vi "Main Controller.vi"(8 "Error In":errorcluster) -> (0 "Error Out":errorcluster)   [LabVIEW 2017, in "Main controller.lvlib"]
uses:
  Main controller.lvlib
  CTLs/Params.ctl
  DAQ/Controls/Params.ctl
  DAQ/Controls/DAQ Config.ctl
  DAQ/Controls/DAQ Indicators.ctl
  CTLs/Test Type.ctl
  Shutter Module/Controls/Params.ctl
  Monochromator/Controls/VISA parameters.ctl
  Monochromator/Controls/Params.ctl
  Monochromator/Controls/Type.ctl
  Monochromator/Controls/GratingValues.ctl
  Monochromator/Controls/Grating.ctl
  Monochromator/PTI/Controls/Params.ctl
  Monochromator/Custom Oriel drivers/Controls/Params.ctl
  C:/Project Work/icl-optical-software-rewrite/Optical Software Code Simplified/Modules/Monochromator/Cornerstone.dll
  Monochromator/Cornerstone.dll
  CTLs/Test params.ctl
  CTLs/Test Controls.ctl
  CTLs/Test indicators.ctl
  Scope/Controls/Params.ctl
  Scope/Controls/Models.ctl
  Scope/Controls/TPC.ctl
  Scope/Controls/Channels.ctl
  Trigger/Controls/Params.ctl
  Trigger/Controls/Mode.ctl
  Trigger/Controls/Trigger channels.ctl
  Scope/Controls/Acquisition type.ctl
  Scope/Controls/Record length.ctl
  Scope/Controls/Data.ctl
  Scope/Controls/Channel data.ctl
  Colour Wheel/Controls/Params.ctl
  File IO/Controls/Params.ctl
  CTLs/Commands [enum].ctl
  Events/Controls/Action Refs [enum].ctl
  Shutter Module/Shutter.lvlib
  Monochromator/Monochromator.lvlib
  UI/UI.lvlib
  DAQ/DAQ.lvlib
  Serial comms/Serial comms.lvlib
  Scope/Scope.lvlib
  Trigger/Trigger.lvlib
  File IO/File IO.lvlib
  Colour Wheel/Colour Wheel.lvlib
  Monochromator/Custom Oriel drivers/Oriel (custom drivers).lvlib
  Monochromator/PTI/PTI.lvlib
  Events/Events.lvlib
  Processing/Processing.lvlib
panel:
  out "Current State":T1
  in  "Commands":T1
  out "Standalone":bool
  out "Config out":T2={"DAQ"={"Data"={"Live"={"t0"=timestamp(0 s since 1904-01-01), "dt"=1.0, "Y"=[]}, "Accumulated"={"t0"=timestamp(0 s since 1904-01-01), "dt"=1.0, "Y"=[]}, "Averaged"={"t0"=timestamp(0 s since 1904-01-01), "dt"=1.0, "Y"=[]}, "data array"=[], "live time array"=[], "Live (decimated)"={"t0"=timestamp(0 s since 1904-01-01), "dt"=1.0, "Y"=[]}}, "Config"={"Input Config"=-1, "Card"=enum."USB-6211", "100% Reflectance Standard (V)"=1.0, "Input Channel"="Dev2/ai0", "Average number of points"=10.0, "Trigger Level (V)"=0.3, "Rate (Hz)"=250000, "End Time (s)"=1.0}, "Indicators"={"Final number of points"=0.0, "Number of samples"=0.0, "dt"=0.0, "Shots"=1, "Shot counter"=0, "Test counter"=0, "Background level (V)"=0.0, "DAQ task"="", "timestamp of data"=timestamp(0 s since 1904-01-01), "Test Type"=enum."A-Test"}}, "Shutter"={"Open command string"="", "VISA"={"Timeout (ms)"=0, "Resource Name"="", "Baud Rate"=0, "Data Bits"=0, "Parity"=0, "Stop Bits"=0, "Flow Control"=0}}, "Monochromator"={"Type"=enum."Oriel", "Wavelength (nm)"=0.0, "Grating, gr/mm"=enum."2400", "Grating mode"=enum."Unknown", "Spectrum mode"={"Spectrum mode?"=FALSE, "Start wavelength (nm)"=0.0, "End wavelength (nm)"=0.0, "Wavelength step (nm)"=0.0, "Wavelength array"=[], "array index"=0}, "PTI"={"Delay before read (ms)"=0, "Mono 1"={"Timeout (ms)"=0, "Resource Name"="", "Baud Rate"=0, "Data Bits"=0, "Parity"=0, "Stop Bits"=0, "Flow Control"=0}, "Mono 2"={"Timeout (ms)"=0, "Resource Name"="", "Baud Rate"=0, "Data Bits"=0, "Parity"=0, "Stop Bits"=0, "Flow Control"=0}, "Two PTI Monochromators?"=FALSE}, "Oriel (custom)"={"reference"=refnum}, "Force wavelength confirmation (PTI)?"=FALSE}, "Test"={"Config"={"Amplification Factor"=0.0, "100% Reflectance Standard"=0.0, "Calculation Method"=enum."Reflectance", "Option to discard new data?"=FALSE, "Mode"=enum."Spectrum", "Number of Averages"=0, "B Test?"=FALSE}, "Indicators"={"DAQ Background Level (V)"=0.0, "A-Test Counter"=0, "B-Test Counter"=0, "Type"=enum."A-Test", "Scope Background Level (Amps)"=2.0, "TAS only?"=FALSE}}, "Scope"={"Config"={"VISA Resource"="USB0::0x0699::0x039D::C010764::INSTR", "Model"=enum."DPO 2012B", "Timebase"=0.0004, "Timeout (ms)"=60000, "TAS"={"Vertical Range (V)"=2.0, "Vertical Offset (0.0 divs)"=0.0, "Bandwidth"=0, "Probe Attenuation (10.0)"=1.0, "Vertical Coupling"=1, "Impedance"=0, "Multiplication factor"=1.0, "Channel"=enum."Channel 1"}, "TPC"={"Vertical Range (V)"=2.0, "Vertical Offset (0.0 divs)"=0.0, "Bandwidth"=0, "Probe Attenuation (10.0)"=1.0, "Vertical Coupling"=1, "Impedance"=0, "Multiplication factor"=1.0, "Channel"=enum."None"}, "Trigger"={"Mode"=enum."Laser (TAS)", "Source "=enum."Aux", "PIA"={"Test LEDs"=FALSE, "LED line"="", "LED off (s)"=0.0, "LED on (s)"=0.0}, "Threshold (V)"=0.8}}, "Indicators"={"Setup"={"Final number of points"=0.0, "Pretrigger points"=0.0, "Number of readouts"=0, "Model"={"Acquisition Type"=4, "Record length (points)"=1000, "Averages on scope"=4, "Average number of points"=10.0}}, "Timestamp of Data"=timestamp(0 s since 1904-01-01)}, "Data"={"TPC"={"Live data"={"t0"=timestamp(0 s since 1904-01-01), "dt"=1.0, "Y"=[]}, "Averaged data"={"t0"=timestamp(0 s since 1904-01-01), "dt"=1.0, "Y"=[]}, "Accumulated data"={"t0"=timestamp(0 s since 1904-01-01), "dt"=1.0, "Y"=[]}, "Final data"={"t0"=timestamp(0 s since 1904-01-01), "dt"=1.0, "Y"=[]}}, "TAS"={"Live data"={"t0"=timestamp(0 s since 1904-01-01), "dt"=1.0, "Y"=[]}, "Averaged data"={"t0"=timestamp(0 s since 1904-01-01), "dt"=1.0, "Y"=[]}, "Accumulated data"={"t0"=timestamp(0 s since 1904-01-01), "dt"=1.0, "Y"=[]}, "Final data"={"t0"=timestamp(0 s since 1904-01-01), "dt"=1.0, "Y"=[]}}, "Time arrays"={"Time array (decimated)"=[], "waveform"={"t0"=timestamp(0 s since 1904-01-01), "dt"=1.0, "Y"=[]}}}, "Test"={"Config"={"Amplification Factor"=0.0, "100% Reflectance Standard"=0.0, "Calculation Method"=enum."Reflectance", "Option to discard new data?"=FALSE, "Mode"=enum."Spectrum", "Number of Averages"=100, "B Test?"=FALSE}, "Indicators"={"DAQ Background Level (V)"=2.0, "A-Test Counter"=2, "B-Test Counter"=2, "Type"=enum."A-Test", "Scope Background Level (Amps)"=2.0, "TAS only?"=FALSE}}}, "Colour wheel"={"Reference"=0, "Colour Wheel Wavelengths"=[], "Waveform Index"=0, "COM Port"="", "Enabled?"=FALSE}, "File IO"={"Output Folder"=path "C:/Users/Abigail/Documents/Imperial Optical software/Optical Software Code Simplified/Output", "Error file"=path "C:/Users/Abigail/Documents/Imperial Optical software/Optical Software Code Simplified/Error Log.txt", "Config file"=path "C:/Users/Abigail/Documents/Imperial Optical software/Optical Software Code Simplified/Config.ini", "File prefix"="", "Waveform read"={"t0"=timestamp(0 s since 1904-01-01), "dt"=1.0, "Y"=[]}}} {"Scope"."Test"."Config"."Number of Averages" min=0; "Scope"."Indicators"."Setup"."Model"."Record length (points)" items=["1000"=1, "10,000"=10, "100,000"=100, "1,000,000"=1000, "5,000,000"=5000, "10,000,000"=10000]; "Scope"."Indicators"."Setup"."Model"."Acquisition Type" items=["Sample", "Peak Detect", "Hi Res", "Envelope", "Average"]; "Scope"."Config"."Trigger"."Threshold (V)" format="%#_3f"; "Scope"."Config"."TPC"."Impedance" items=["1M", "75", "50"]; "Scope"."Config"."TPC"."Vertical Coupling" items=["AC", "DC", "Ground"]; "Scope"."Config"."TPC"."Bandwidth" items=["FULL", "250 MHz", "150 MHz", "20 MHz"]; "Scope"."Config"."TAS"."Impedance" items=["1M", "75", "50"]; "Scope"."Config"."TAS"."Vertical Coupling" items=["AC", "DC", "Ground"]; "Scope"."Config"."TAS"."Bandwidth" items=["FULL", "250 MHz", "150 MHz", "20 MHz"]; "Scope"."Config"."Timebase" format="%^#_3e"; "Test"."Config"."Number of Averages" min=0; "Monochromator"."PTI"."Mono 2"."Flow Control" items=["1.0"=10, "1.5"=15, "2.0"=20]; "Monochromator"."PTI"."Mono 2"."Stop Bits" items=["None", "Odd", "Even", "Mark", "Space"]; "Monochromator"."PTI"."Mono 2"."Parity" items=["None", "Odd", "Even", "Mark", "Space"]; "Monochromator"."PTI"."Mono 1"."Flow Control" items=["1.0"=10, "1.5"=15, "2.0"=20]; "Monochromator"."PTI"."Mono 1"."Stop Bits" items=["None", "Odd", "Even", "Mark", "Space"]; "Monochromator"."PTI"."Mono 1"."Parity" items=["None", "Odd", "Even", "Mark", "Space"]; "Shutter"."VISA"."Flow Control" items=["None"=0, "XON/XOFF"=1, "RTS/CTS"=2, "DTR/DSR"=4]; "Shutter"."VISA"."Stop Bits" items=["1.0"=10, "1.5"=15, "2.0"=20]; "Shutter"."VISA"."Parity" items=["None", "Odd", "Even", "Mark", "Space"]; "DAQ"."Config"."Input Config" items=["default"=-1, "RSE"=10083, "NRSE"=10078, "Differential"=10106, "Pseudodifferential"=12529]}
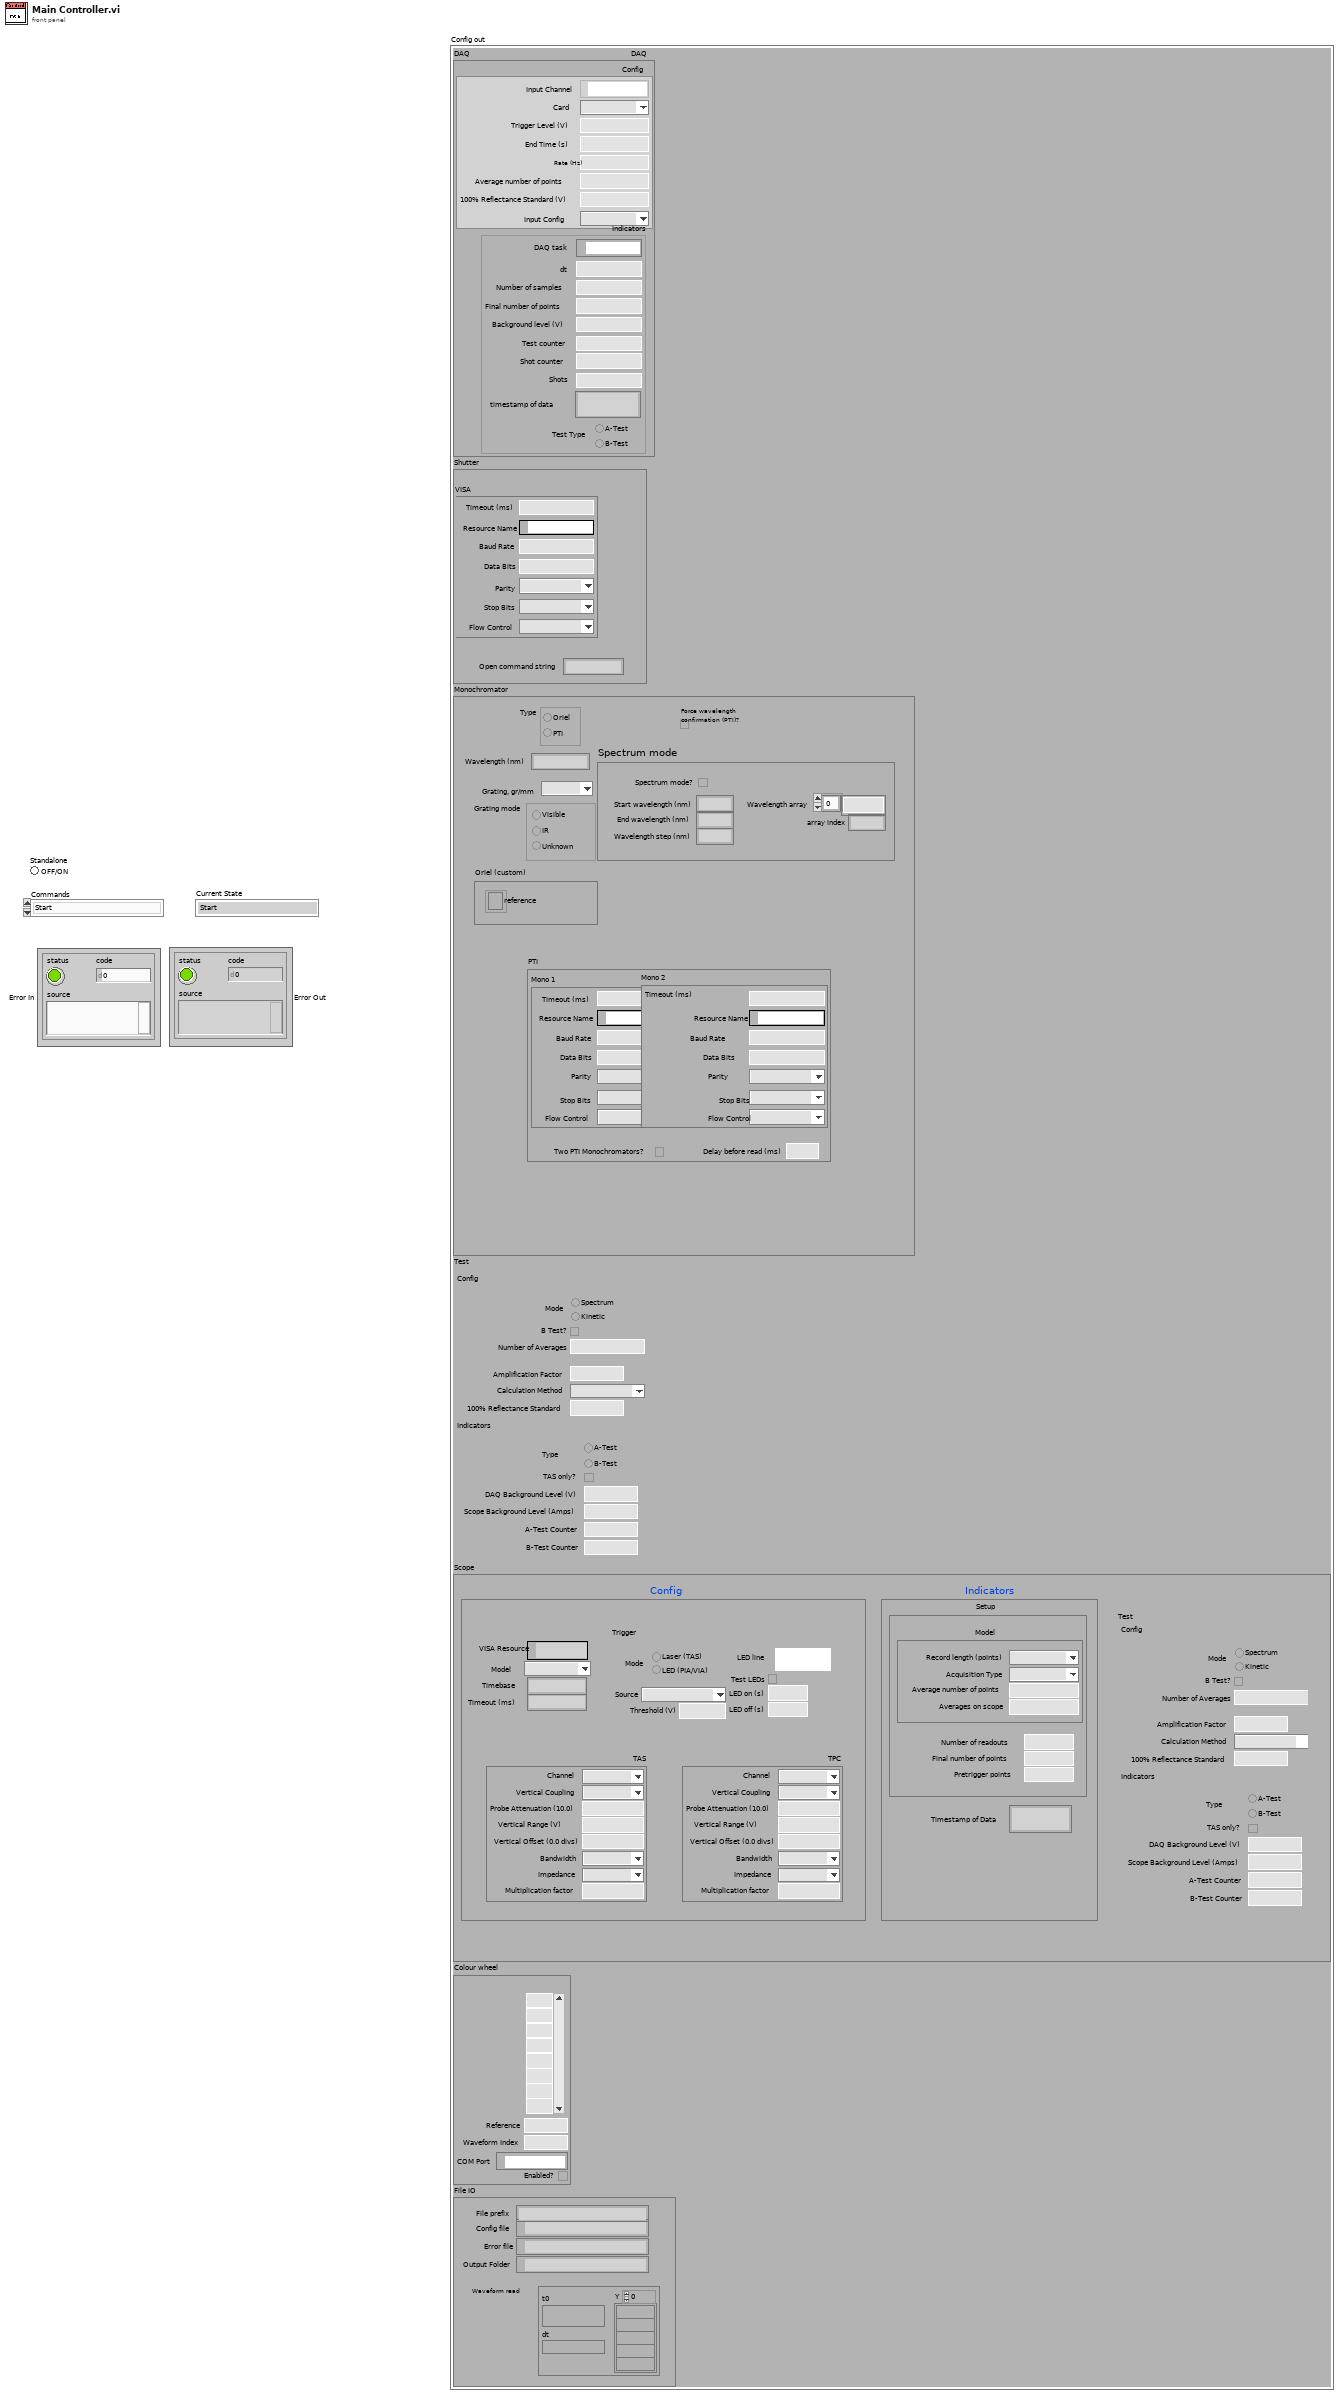
[diagram p1: front panel]
types:
  T1 = typedef "Main controller.lvlib/Commands [enum].ctl" = enum16{"Start", "Initialise Devices", "Stop", "Set DAQ data", "Set Scope data", "Set Spectrum Setup", "Spectrum Setup Complete", "Set Monochromator Setup", "Monochromator Setup Complete", "Set Monochromator data", "Set Colour Wheel Setup", "Colour Wheel Setup Complete", "Move Shutter", "Move Shutter Complete", "Collect Data", "DAQ Acquisition Complete", "Scope Acquisition Complete", "Collect Data Complete", "A-B Processing", "A-B Processing Complete", "DAQ-Scope Stitching", "DAQ-Scope Stitching Complete", "Return Shutter", "Return Shutter Complete", "Set colour wheel data", "Set all config data", "Acquire test data", "Accumulate test data", "Average test data", "All Averaging Complete", "DAQ Averaging Complete", "Scope Averaging Complete", "Finalise test data", "All Finalising Complete", "DAQ Finalising Complete", "Scope Finalising Complete", "Process test data", "End Test"}
  T2 = typedef "Main controller.lvlib/Params.ctl" = cluster{"DAQ":T3, "Shutter":T7, "Monochromator":T9, "Test":T15, "Scope":T18, "Colour wheel":T29, "File IO":T30}
  T3 = typedef "DAQ.lvlib/Params.ctl" = cluster{"Data":cluster{"Live":waveform(dbl), "Accumulated":waveform(dbl), "Averaged":waveform(dbl), "data array":dbl[], "live time array":dbl[], "Live (decimated)":waveform(dbl)}, "Config":T4, "Indicators":T5}
  T4 = typedef "DAQ.lvlib/DAQ Config.ctl" = cluster{"Input Config":i32, "Card":enum16{"USB-6211", "USB-6251", "USB-6361"}, "100% Reflectance Standard (V)":dbl, "Input Channel":tag, "Average number of points":dbl, "Trigger Level (V)":dbl, "Rate (Hz)":i32, "End Time (s)":dbl}
  T5 = typedef "DAQ.lvlib/DAQ Indicators.ctl" = cluster{"Final number of points":dbl, "Number of samples":dbl, "dt":dbl, "Shots":i32, "Shot counter":i32, "Test counter":i32, "Background level (V)":dbl, "DAQ task":refnum<k21>, "timestamp of data":timestamp, "Test Type":T6}
  T6 = typedef "Main controller.lvlib/Test Type.ctl" = enum32{"A-Test", "B-Test"}
  T7 = typedef "Shutter.lvlib/Params.ctl" = cluster{"Open command string":string, "VISA":T8}
  T8 = typedef "Serial comms.lvlib/VISA parameters.ctl" = cluster{"Timeout (ms)":u32, "Resource Name":refnum<visa-resource-name>, "Baud Rate":u32, "Data Bits":u16, "Parity":u16, "Stop Bits":u16, "Flow Control":u16}
  T9 = typedef "Monochromator.lvlib/Params.ctl" = cluster{"Type":T10, "Wavelength (nm)":dbl, "Grating, gr/mm":T11, "Grating mode":T12, "Spectrum mode":cluster{"Spectrum mode?":bool, "Start wavelength (nm)":dbl, "End wavelength (nm)":dbl, "Wavelength step (nm)":dbl, "Wavelength array":dbl[], "array index":u32}, "PTI":T13, "Oriel (custom)":T14, "Force wavelength confirmation (PTI)?":bool}
  T10 = typedef "Monochromator.lvlib/Type.ctl" = enum32{"Oriel", "PTI"}
  T11 = typedef "Monochromator.lvlib/GratingValues.ctl" = enum16{"2400", "1800", "1200", "600", "300", "150"}
  T12 = typedef "Monochromator.lvlib/Grating.ctl" = enum32{"Unknown", "Visible", "IR"}
  T13 = typedef "Monochromator.lvlib/PTI.lvlib/Params.ctl" = cluster{"Delay before read (ms)":u32, "Mono 1":T8, "Mono 2":T8, "Two PTI Monochromators?":bool}
  T14 = typedef "Monochromator.lvlib/Oriel (custom drivers).lvlib/Params.ctl" = cluster{"reference":refnum<k24>}
  T15 = typedef "Main controller.lvlib/Test params.ctl" = cluster{"Config":T16, "Indicators":T17}
  T16 = typedef "Main controller.lvlib/Test Controls.ctl" = cluster{"Amplification Factor":dbl, "100% Reflectance Standard":dbl, "Calculation Method":enum16{"Reflectance", "Transmission", "Kubelka-Munk"}, "Option to discard new data?":bool, "Mode":enum32{"Spectrum", "Kinetic"}, "Number of Averages":i32, "B Test?":bool}
  T17 = typedef "Main controller.lvlib/Test indicators.ctl" = cluster{"DAQ Background Level (V)":dbl, "A-Test Counter":i32, "B-Test Counter":i32, "Type":T6, "Scope Background Level (Amps)":dbl, "TAS only?":bool}
  T18 = typedef "Scope.lvlib/Params.ctl" = cluster{"Config":cluster{"VISA Resource":refnum<visa-resource-name>, "Model":T19, "Timebase":dbl, "Timeout (ms)":u32, "TAS":T20, "TPC":T20, "Trigger":T22}, "Indicators":cluster{"Setup":cluster{"Final number of points":dbl, "Pretrigger points":dbl, "Number of readouts":i32, "Model":cluster{"Acquisition Type":T25, "Record length (points)":T26, "Averages on scope":i32, "Average number of points":dbl}}, "Timestamp of Data":timestamp}, "Data":T27, "Test":T15}
  T19 = typedef "Scope.lvlib/Models.ctl" = enum16{"DPO 3012", "DPO 2012B", "TDS 3012C"}
  T20 = typedef "Scope.lvlib/TPC.ctl" = cluster{"Vertical Range (V)":dbl, "Vertical Offset (0.0 divs)":dbl, "Bandwidth":i32, "Probe Attenuation (10.0)":dbl, "Vertical Coupling":u16, "Impedance":u16, "Multiplication factor":dbl, "Channel":T21}
  T21 = typedef "Scope.lvlib/Channels.ctl" = enum16{"Channel 1", "Channel 2", "Channel 3", "Channel 4", "Math", "Reference A", "Reference B", "Reference C", "Reference D", "B1", "B2", "None"}
  T22 = typedef "Scope.lvlib/Trigger.lvlib/Params.ctl" = cluster{"Mode":T23, "Source ":T24, "PIA":cluster{"Test LEDs":bool, "LED line":tag, "LED off (s)":dbl, "LED on (s)":dbl}, "Threshold (V)":dbl}
  T23 = typedef "Scope.lvlib/Trigger.lvlib/Mode.ctl" = enum32{"Laser (TAS)", "LED (PIA/VIA)"}
  T24 = typedef "Scope.lvlib/Trigger.lvlib/Trigger channels.ctl" = enum16{"Channel 1", "Channel 2", "Channel 3", "Channel 4", "AC Line", "Aux", "Digital Channel 0", "Digital Channel 1", "Digital Channel 2", "Digital Channel 3", "Digital Channel 4", "Digital Channel 5", "Digital Channel 6", "Digital Channel 7", "Digital Channel 8", "Digital Channel 9", "Digital Channel 10", "Digital Channel 11", "Digital Channel 12", "Digital Channel 13", "Digital Channel 14", "Digital Channel 15", "RF"}
  T25 = typedef "Scope.lvlib/Acquisition type.ctl" = u16
  T26 = typedef "Scope.lvlib/Record length.ctl" = u32
  T27 = typedef "Scope.lvlib/Data.ctl" = cluster{"TPC":T28, "TAS":T28, "Time arrays":cluster{"Time array (decimated)":dbl[], "waveform":waveform(dbl)}}
  T28 = typedef "Scope.lvlib/Channel data.ctl" = cluster{"Live data":waveform(dbl), "Averaged data":waveform(dbl), "Accumulated data":waveform(dbl), "Final data":waveform(dbl)}
  T29 = typedef "Colour Wheel.lvlib/Params.ctl" = cluster{"Reference":i32, "Colour Wheel Wavelengths":dbl[], "Waveform Index":i32, "COM Port":refnum<visa-resource-name>, "Enabled?":bool}
  T30 = typedef "File IO.lvlib/Params.ctl" = cluster{"Output Folder":path, "Error file":path, "Config file":path, "File prefix":string, "Waveform read":waveform(dbl)}
  T31 = cluster{"DAQ Acq Complete":bool, "Scope Acq Complete":bool, "DAQ Average Complete":bool, "Scope Average Complete":bool, "DAQ Finalising Complete":bool, "Scope Finalising Complete":bool, "Test Complete":bool}
  T32 = enum32{"Bad", "Idle", "Run top level", "Running"}
  T33 = typedef "Events.lvlib/Action Refs [enum].ctl" = enum16{"Init", "Ref", "Kill"}
  T34 = typedef "Events.lvlib/Refs [cluster].ctl" = cluster{"Exit":refnum<user-event>, "Controller":refnum<user-event>, "System Error":refnum<user-event>, "UI":refnum<user-event>, "Example Module":refnum<user-event>, "Shutter":refnum<user-event>, "Monochromator":refnum<user-event>, "DAQ":refnum<user-event>, "Scope":refnum<user-event>, "Processing":refnum<user-event>, "File IO":refnum<user-event>, "Colour wheel":refnum<user-event>}
  T35 = cluster{"Live":waveform(dbl), "Accumulated":waveform(dbl), "Averaged":waveform(dbl), "data array":dbl[], "live time array":dbl[], "Live (decimated)":waveform(dbl)}
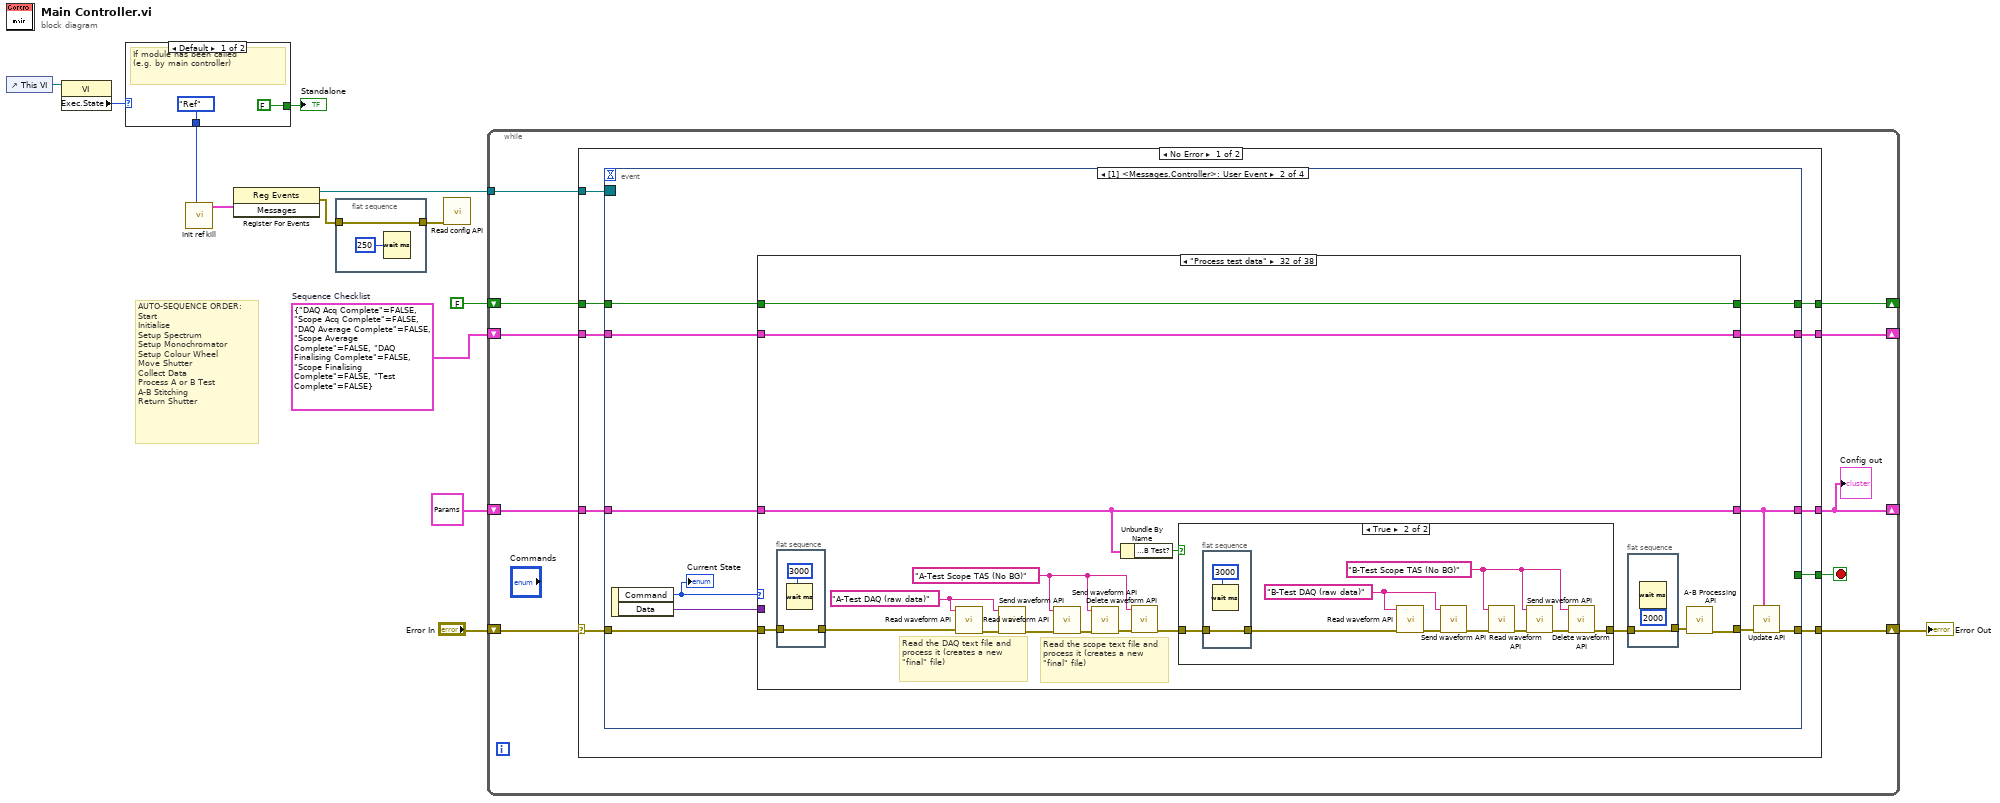
[diagram p0: block diagram]
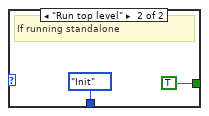
[diagram p2: hidden frame]
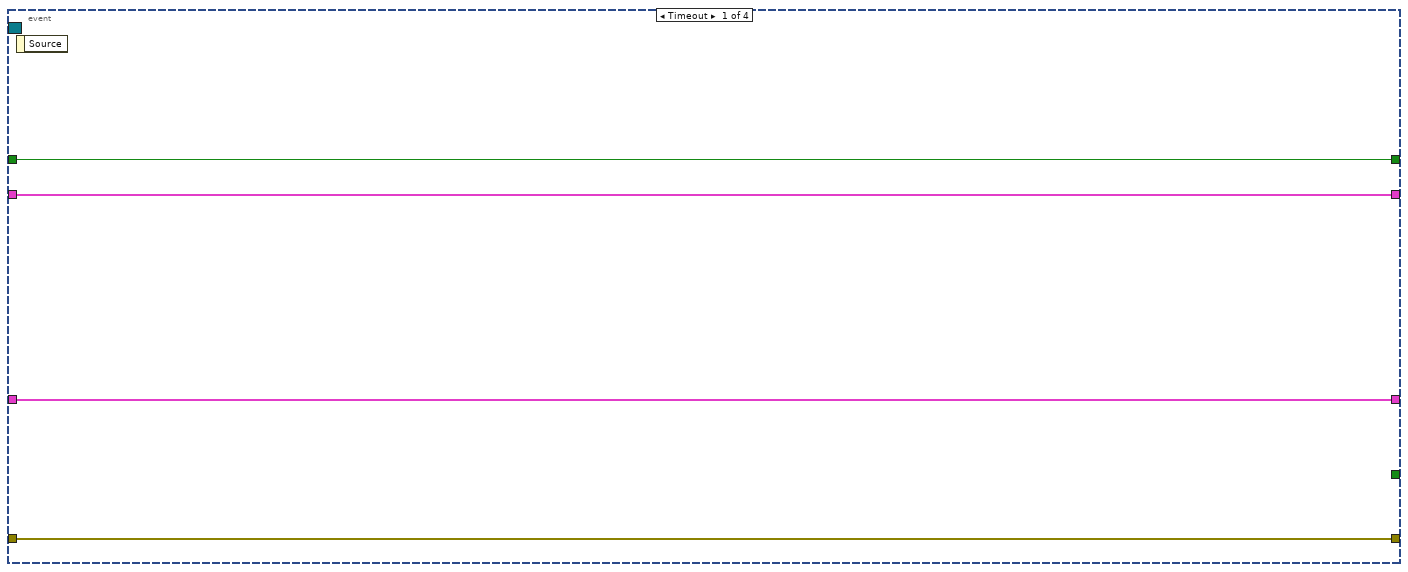
[diagram p3: hidden frame]
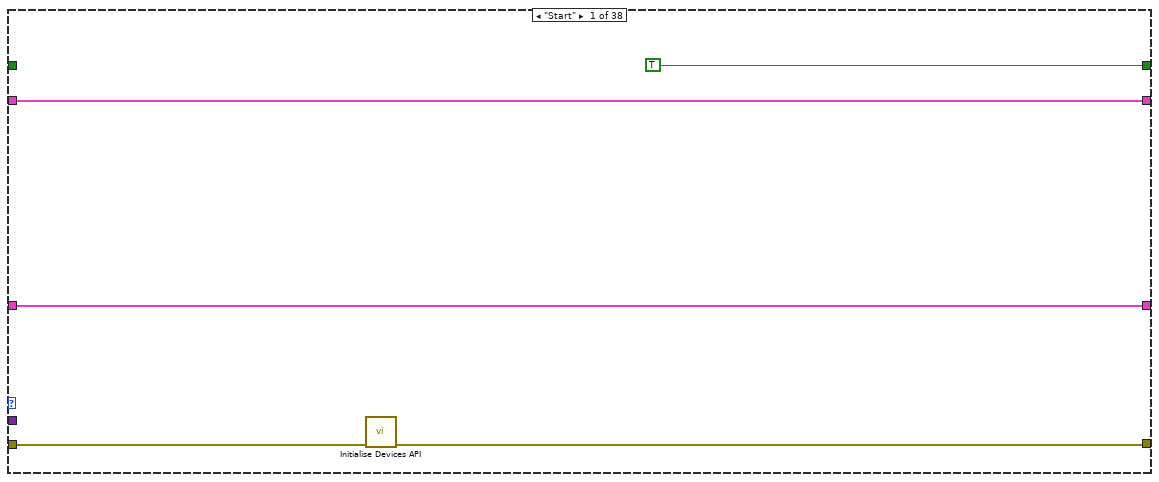
[diagram p4: hidden frame]
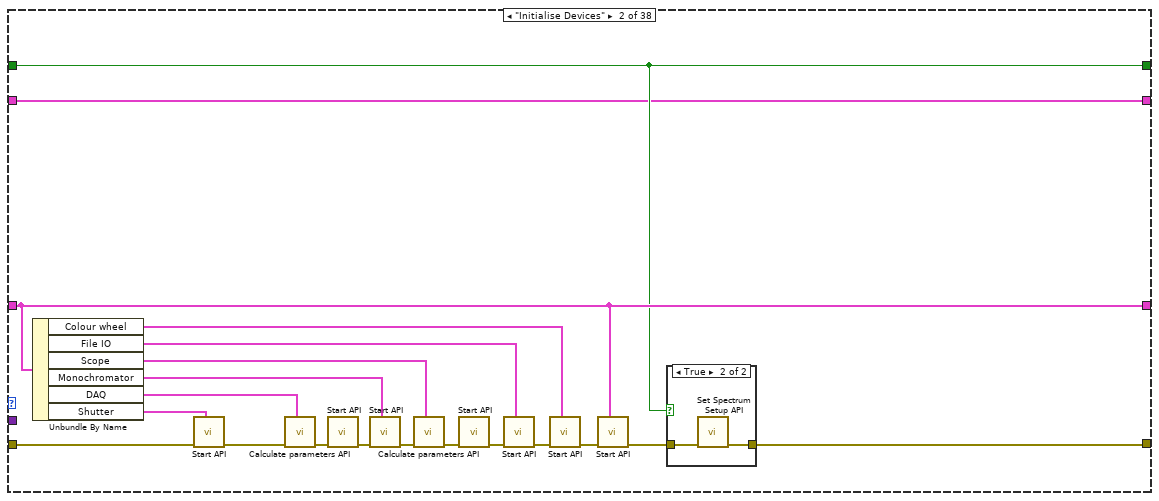
[diagram p5: hidden frame]
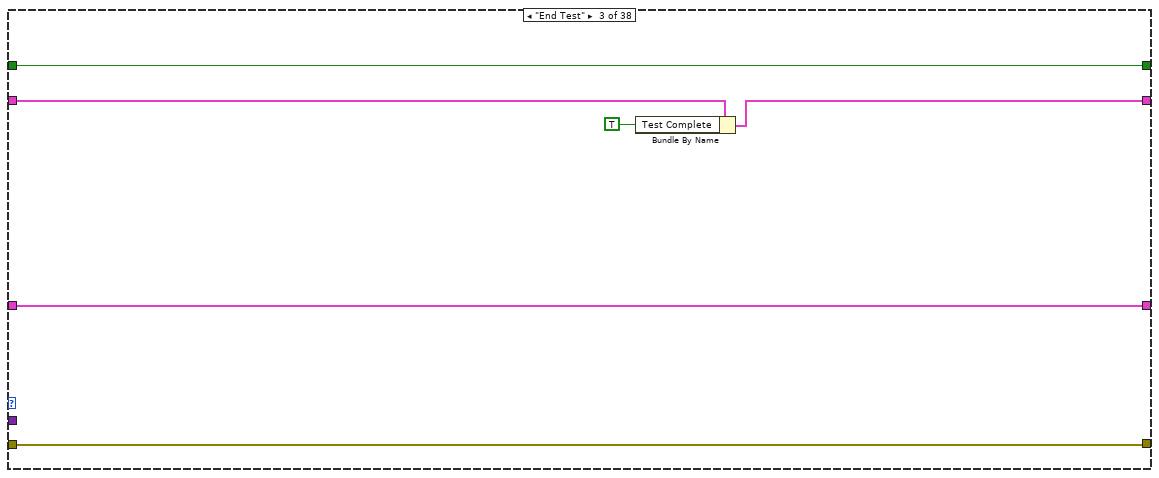
[diagram p7: hidden frame]
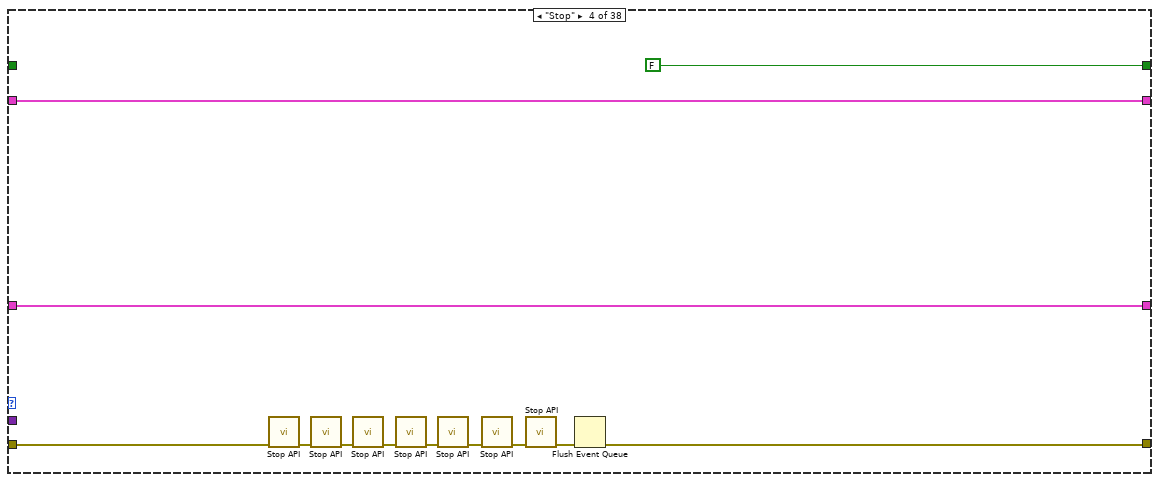
[diagram p8: hidden frame]
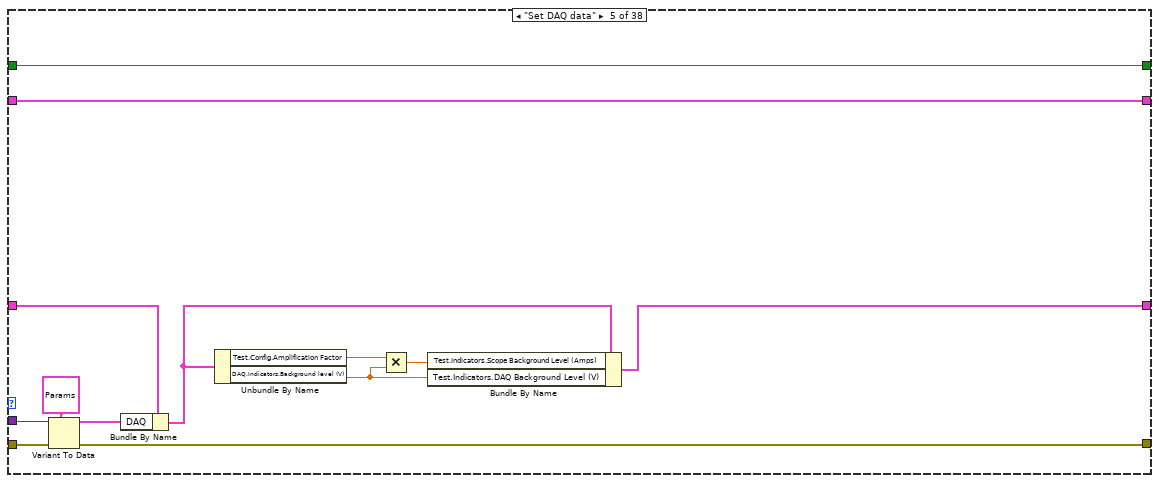
[diagram p9: hidden frame]
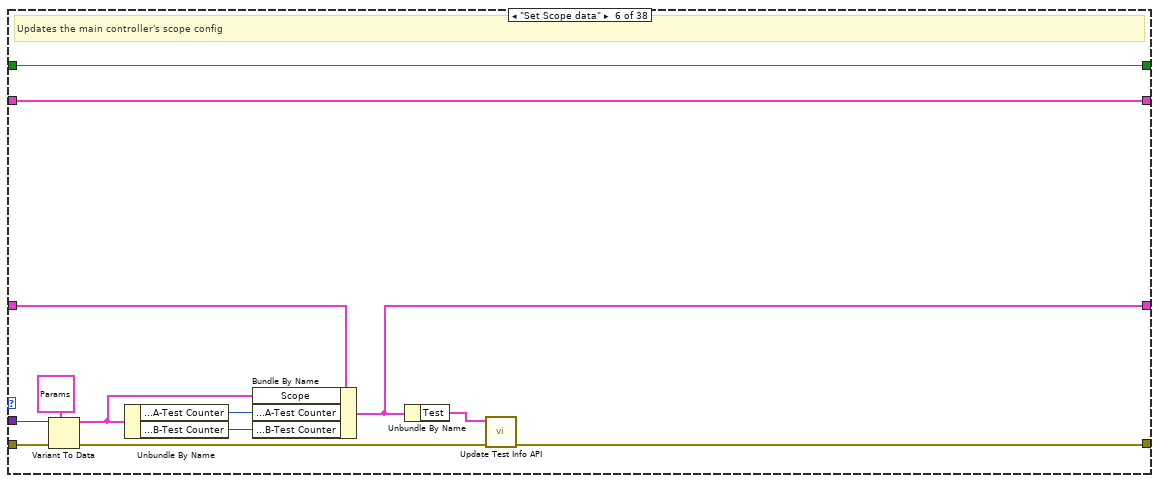
[diagram p10: hidden frame]
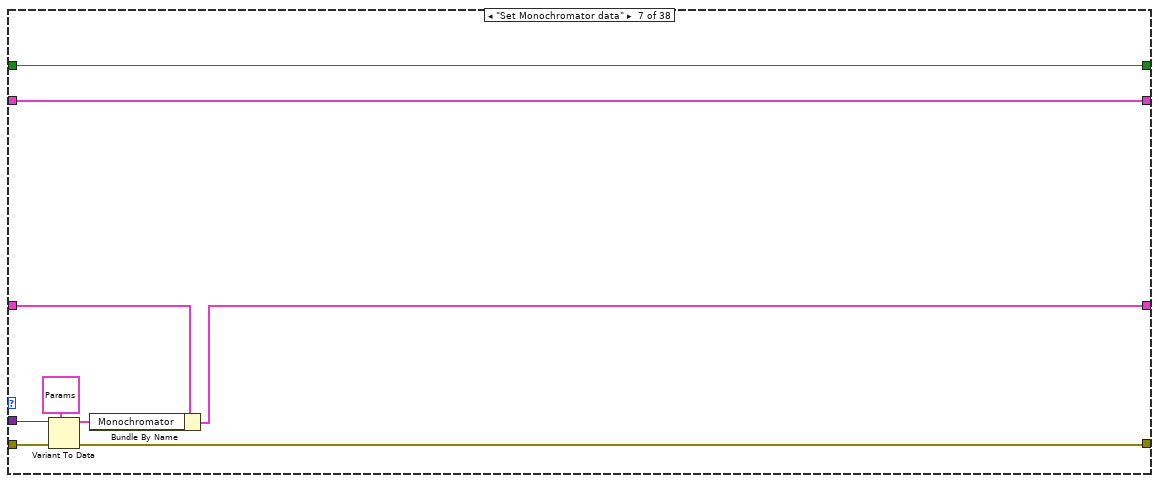
[diagram p11: hidden frame]
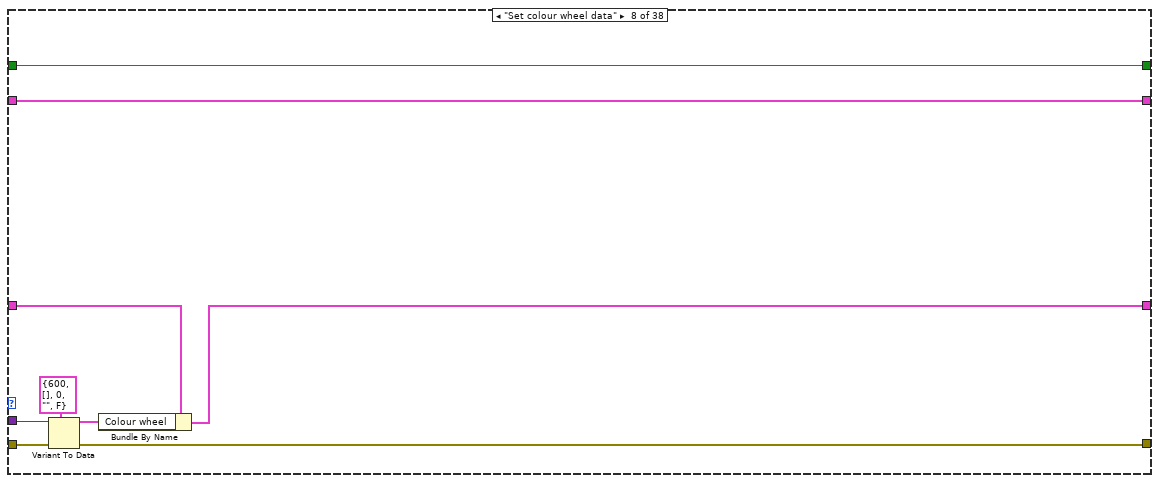
[diagram p12: hidden frame]
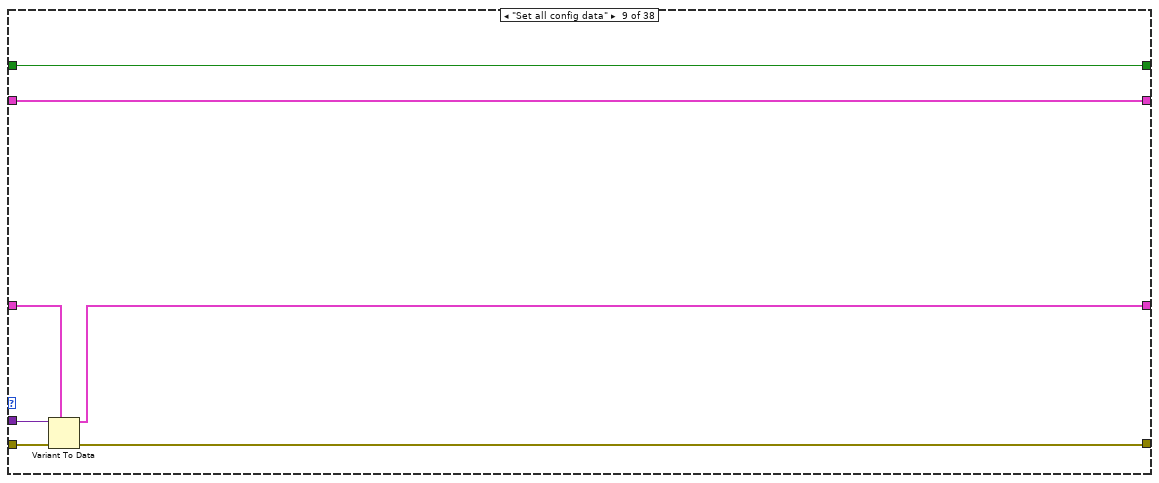
[diagram p13: hidden frame]
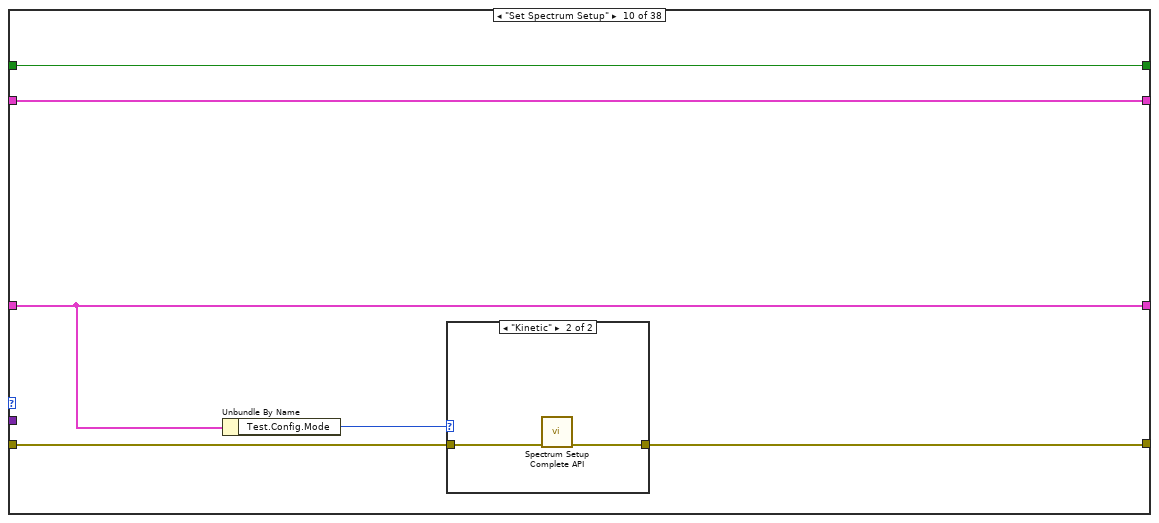
[diagram p14: hidden frame]
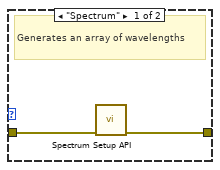
[diagram p15: hidden frame]
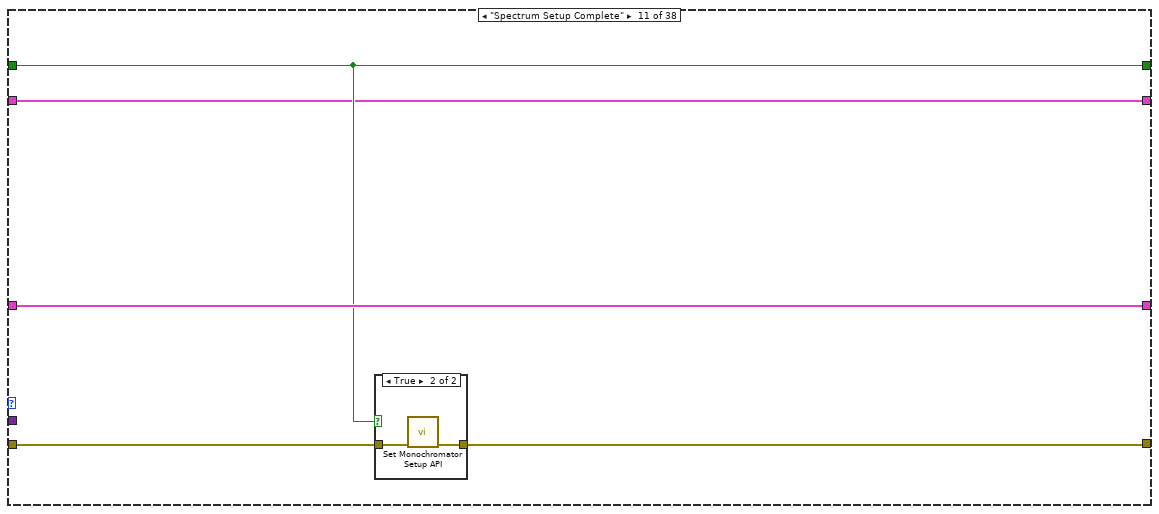
[diagram p16: hidden frame]
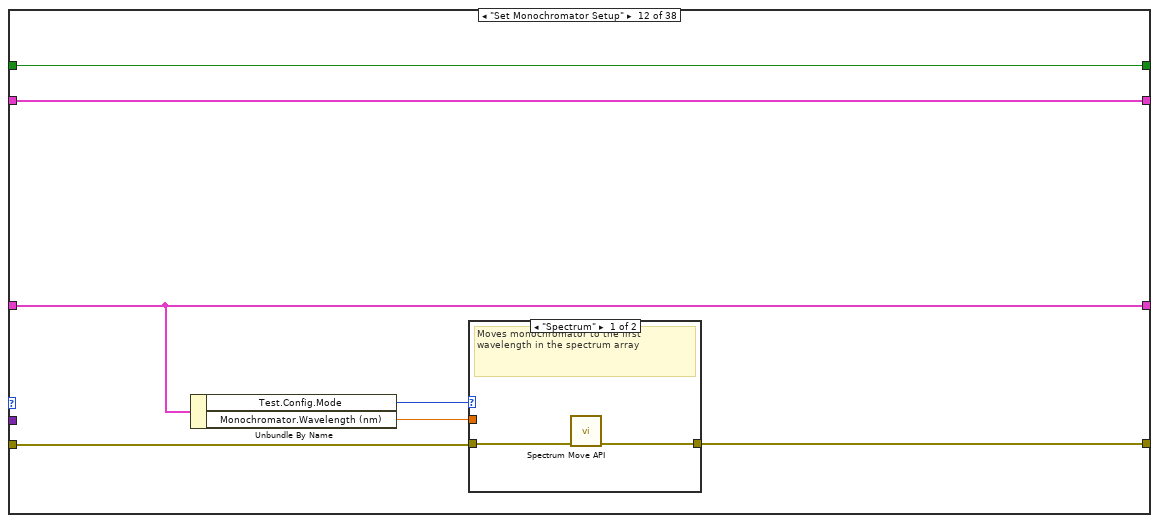
[diagram p18: hidden frame]
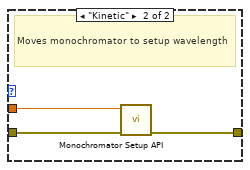
[diagram p19: hidden frame]
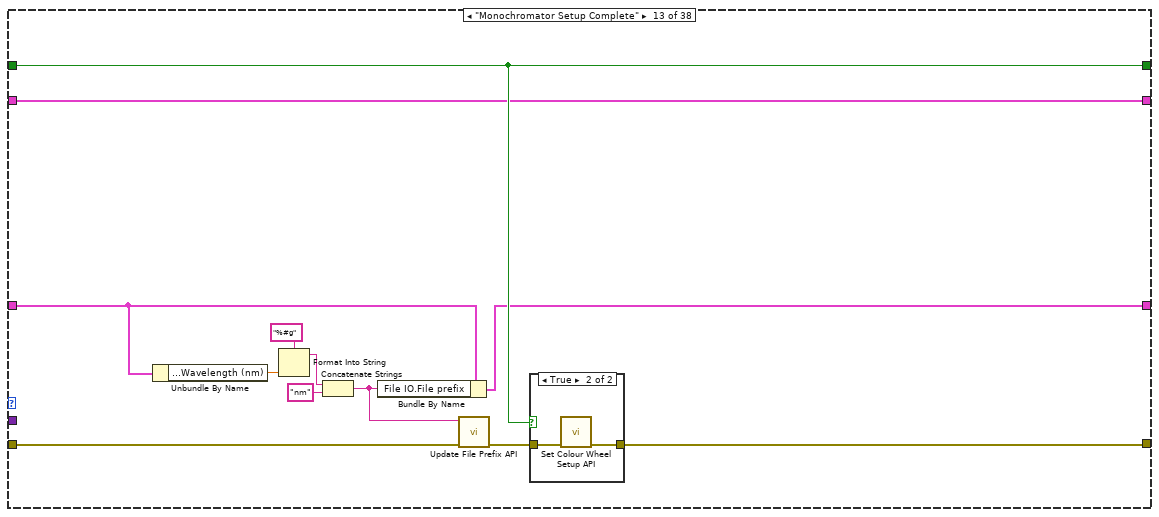
[diagram p20: hidden frame]
diagram:
  w1 = T31 {"DAQ Acq Complete"=FALSE, "Scope Acq Complete"=FALSE, "DAQ Average Complete"=FALSE, "Scope Average Complete"=FALSE, "DAQ Finalising Complete"=FALSE, "Scope Finalising Complete"=FALSE, "Test Complete"=FALSE}  # Sequence Checklist
  # "AUTO-SEQUENCE ORDER:\nStart\nInitialise\nSetup Spectrum\nSetup Monochromator\nSetup Colour Wheel\nMove Shutter\nCollect Data\nProcess A or B Test\nA-B Stitching\nReturn Shutter"
  n1 = control-ref of="This VI"() -> (w11:refnum<vi>)
  n2 = property class="VI"(reference=w11) -> ("Exec.State"=w10:T32)  [unwired: 1 in, 2 out]
  n3 = case shown="Default" w10 {
    tunnel: [Action_Refs_[enum]."Ref" ("Action") Action_Refs_[enum]."Init" ("Action")] -> w9
    tunnel: [FALSE TRUE] -> w8
    frame Default {
      # "If module has been called\n(e.g. by main controller)"
    }
    frame "Run top level" {
      # "If running standalone"
    }
  }
  "Standalone" <- w8
  n4 = call "Init ref kill.vi"("Action"=w9) -> ("Messages"=w5:T34)  [unwired: 9 in, 1 out]
  n5 = register-events(w5) -> (reference out=w4:refnum<event-registration>, error out=w3:errorcluster)  [unwired: 2 in]
  n6 = flat-sequence {
    tunnel: w3 -> [w19]
    tunnel: [w19] -> w2
    frame #0 {
      n7 = Wait (ms)(milliseconds to wait=u32 250) -> ()  [unwired: 1 out]
    }
  }
  n8 = call "Read config API.vi"("Error In"=w2) -> ()  [unwired: 10 in, 1 out]
  n9 = while {
    shift-right: [w29] -> w12
    shift-left: "Error In" -> [w24]
    shift-right: [w26] -> _
    shift-left: T2 {"DAQ"={"Data"={"Live"={"t0"=timestamp(0 s since 1904-01-01), "dt"=1.0, "Y"=[]}, "Accumulated"={"t0"=timestamp(0 s since 1904-01-01), "dt"=1.0, "Y"=[]}, "Averaged"={"t0"=timestamp(0 s since 1904-01-01), "dt"=1.0, "Y"=[]}, "data array"=[], "live time array"=[], "Live (decimated)"={"t0"=timestamp(0 s since 1904-01-01), "dt"=1.0, "Y"=[]}}, "Config"={"Input Config"=10106, "Card"=enum."USB-6211", "100% Reflectance Standard (V)"=1.0, "Input Channel"="Dev1/ai0", "Average number of points"=50.0, "Trigger Level (V)"=0.4, "Rate (Hz)"=250000, "End Time (s)"=1.0}, "Indicators"={"Final number of points"=0.0, "Number of samples"=0.0, "dt"=0.0, "Shots"=1, "Shot counter"=0, "Test counter"=0, "Background level (V)"=0.0, "DAQ task"="", "timestamp of data"=timestamp(0 s since 1904-01-01), "Test Type"=enum."A-Test"}}, "Shutter"={"Open command string"="", "VISA"={"Timeout (ms)"=0, "Resource Name"="", "Baud Rate"=0, "Data Bits"=0, "Parity"=0, "Stop Bits"=0, "Flow Control"=0}}, "Monochromator"={"Type"=enum."Oriel", "Wavelength (nm)"=0.0, "Grating, gr/mm"=enum."2400", "Grating mode"=enum."Unknown", "Spectrum mode"={"Spectrum mode?"=FALSE, "Start wavelength (nm)"=0.0, "End wavelength (nm)"=0.0, "Wavelength step (nm)"=0.0, "Wavelength array"=[], "array index"=0}, "PTI"={"Delay before read (ms)"=0, "Mono 1"={"Timeout (ms)"=0, "Resource Name"="", "Baud Rate"=0, "Data Bits"=0, "Parity"=0, "Stop Bits"=0, "Flow Control"=0}, "Mono 2"={"Timeout (ms)"=0, "Resource Name"="", "Baud Rate"=0, "Data Bits"=0, "Parity"=0, "Stop Bits"=0, "Flow Control"=0}, "Two PTI Monochromators?"=FALSE}, "Oriel (custom)"={"reference"=refnum}, "Force wavelength confirmation (PTI)?"=FALSE}, "Test"={"Config"={"Amplification Factor"=0.0, "100% Reflectance Standard"=0.0, "Calculation Method"=enum."Reflectance", "Option to discard new data?"=FALSE, "Mode"=enum."Spectrum", "Number of Averages"=0, "B Test?"=FALSE}, "Indicators"={"DAQ Background Level (V)"=0.0, "A-Test Counter"=0, "B-Test Counter"=0, "Type"=enum."A-Test", "Scope Background Level (Amps)"=2.0, "TAS only?"=FALSE}}, "Scope"={"Config"={"VISA Resource"="USB0::0x0699::0x039D::C010764::INSTR", "Model"=enum."DPO 2012B", "Timebase"=0.0004, "Timeout (ms)"=60000, "TAS"={"Vertical Range (V)"=2.0, "Vertical Offset (0.0 divs)"=0.0, "Bandwidth"=0, "Probe Attenuation (10.0)"=1.0, "Vertical Coupling"=1, "Impedance"=0, "Multiplication factor"=1.0, "Channel"=enum."Channel 1"}, "TPC"={"Vertical Range (V)"=2.0, "Vertical Offset (0.0 divs)"=0.0, "Bandwidth"=0, "Probe Attenuation (10.0)"=1.0, "Vertical Coupling"=1, "Impedance"=0, "Multiplication factor"=1.0, "Channel"=enum."None"}, "Trigger"={"Mode"=enum."Laser (TAS)", "Source "=enum."Aux", "PIA"={"Test LEDs"=FALSE, "LED line"="", "LED off (s)"=0.0, "LED on (s)"=0.0}, "Threshold (V)"=0.8}}, "Indicators"={"Setup"={"Final number of points"=0.0, "Pretrigger points"=0.0, "Number of readouts"=0, "Model"={"Acquisition Type"=4, "Record length (points)"=1000, "Averages on scope"=4, "Average number of points"=10.0}}, "Timestamp of Data"=timestamp(0 s since 1904-01-01)}, "Data"={"TPC"={"Live data"={"t0"=timestamp(0 s since 1904-01-01), "dt"=1.0, "Y"=[]}, "Averaged data"={"t0"=timestamp(0 s since 1904-01-01), "dt"=1.0, "Y"=[]}, "Accumulated data"={"t0"=timestamp(0 s since 1904-01-01), "dt"=1.0, "Y"=[]}, "Final data"={"t0"=timestamp(0 s since 1904-01-01), "dt"=1.0, "Y"=[]}}, "TAS"={"Live data"={"t0"=timestamp(0 s since 1904-01-01), "dt"=1.0, "Y"=[]}, "Averaged data"={"t0"=timestamp(0 s since 1904-01-01), "dt"=1.0, "Y"=[]}, "Accumulated data"={"t0"=timestamp(0 s since 1904-01-01), "dt"=1.0, "Y"=[]}, "Final data"={"t0"=timestamp(0 s since 1904-01-01), "dt"=1.0, "Y"=[]}}, "Time arrays"={"Time array (decimated)"=[], "waveform"={"t0"=timestamp(0 s since 1904-01-01), "dt"=1.0, "Y"=[]}}}, "Test"={"Config"={"Amplification Factor"=0.0, "100% Reflectance Standard"=0.0, "Calculation Method"=enum."Reflectance", "Option to discard new data?"=FALSE, "Mode"=enum."Spectrum", "Number of Averages"=100, "B Test?"=FALSE}, "Indicators"={"DAQ Background Level (V)"=0.0, "A-Test Counter"=0, "B-Test Counter"=0, "Type"=enum."A-Test", "Scope Background Level (Amps)"=0.0, "TAS only?"=FALSE}}}, "Colour wheel"={"Reference"=0, "Colour Wheel Wavelengths"=[], "Waveform Index"=0, "COM Port"="", "Enabled?"=FALSE}, "File IO"={"Output Folder"=path "C:/Users/Abigail/Documents/Imperial Optical software/Optical Software Code Simplified/Output", "Error file"=path "C:/Users/Abigail/Documents/Imperial Optical software/Optical Software Code Simplified/Error Log.txt", "Config file"=path "C:/Users/Abigail/Documents/Imperial Optical software/Optical Software Code Simplified/Config.ini", "File prefix"="", "Waveform read"={"t0"=timestamp(0 s since 1904-01-01), "dt"=1.0, "Y"=[]}}} ("Config") -> [w27]
    tunnel: w4 -> [w25]
    shift-right: [w22] -> _
    shift-left: FALSE -> [w23]
    shift-right: [w20] -> _
    shift-left: w1 -> [w21]
    stop <- w28 stop-if-true
    n10 = case shown="No Error" w24 {
      selector: w24 -> [w34 w661]
      tunnel: [w39 w660] -> w29
      tunnel: [w38 _] -> w28
      tunnel: w27 -> [w37 w662]
      tunnel: [w36 w662] -> w26
      tunnel: w25 -> [w35 _]
      tunnel: w23 -> [w33 w658]
      tunnel: [w32 w658] -> w22
      tunnel: w21 -> [w31 w657]
      tunnel: [w30 w657] -> w20
      frame No Error {
        n11 = event shown="[1] <Messages.Controller>: User Event" {
          selector: w35 -> [_ _ _ _]
          dyn-events: _ -> [_ _ _ _]
          timeout: _ -> [_ _ _ _]
          tunnel: [w43 w49 w591 w656] -> w39
          tunnel: w34 -> [w43 w54 w590 w656]
          tunnel: [_ _ _ TRUE] -> w38
          tunnel: w37 -> [w42 w51 w588 w654]
          tunnel: [w42 w50 w588 w654] -> w36
          tunnel: w33 -> [w41 w48 w587 w653]
          tunnel: [w41 w47 w587 w653] -> w32
          tunnel: w31 -> [w40 w45 w586 w652]
          tunnel: [w40 w44 w586 w652] -> w30
          event Timeout {
            n12 = event-data() -> ()  [unwired: 1 in, 1 out]
          }
          event User Event {
            n13 = event-data() -> ("Command"=w53:T1, "Data"=w52:variant)  [unwired: 1 in]
            "Current State" <- w53
            n14 = case shown="\"Process test data\"" w53 {
              tunnel: w54 -> [w57 w64 w88 w98 w113 w126 w135 w144 w151 w155 w165 w171 w189 w202 w209 w215 w235 w248 w274 w279 w295 w309 w317 w328 w338 w352 w358 w365 w382 w396 w407 w434 w467 w491 w500 w512 w521 w535]
              tunnel: [w56 w62 w88 w89 w108 w119 w129 w138 w149 w154 w164 w173 w193 w204 w208 w216 w231 w247 w275 w283 w295 w309 w316 w325 w338 w352 w357 w366 w382 w396 w404 w445 w468 w490 w499 w511 w520 w534] -> w46
              tunnel: w52 -> [_ _ _ _ w112 w125 w134 w143 w150 _ _ _ _ _ _ _ _ _ _ _ _ _ _ _ _ _ _ _ _ _ _ _ _ _ _ _ _ _]
              tunnel: w51 -> [w58 w65 w83 w97 w109 w124 w132 w141 w147 w153 w166 w170 w187 w198 w210 w217 w232 w245 w270 w280 w294 w308 w318 w322 w337 w351 w361 w367 w381 w395 w409 w436 w469 w492 w498 w514 w519 w530]
              tunnel: [w58 w65 w83 w97 w103 w117 w131 w140 w148 w153 w166 w170 w186 w198 w210 w217 w232 w246 w270 w280 w294 w308 w318 w322 w337 w351 w361 w367 w381 w395 w408 w436 w469 w492 w498 w514 w519 w529] -> w50
              tunnel: w48 -> [_ w61 w87 _ w107 w122 w128 w137 w146 w157 w163 w176 w192 w205 w207 w220 w234 w250 w272 w282 w293 w307 w315 w324 w336 w350 w360 w370 w380 w394 w411 w444 w471 w489 w502 w510 w523 _]
              tunnel: [TRUE w61 w87 FALSE w107 w122 w128 w137 w146 w157 w163 w176 w192 w205 w207 w220 w234 w250 w272 w282 w293 w307 w315 w324 w336 w350 w360 w370 w380 w394 w411 w444 w471 w489 w502 w510 w523 w531] -> w47
              tunnel: w45 -> [w55 w60 w86 w91 w106 w121 w127 w136 w145 w152 w162 w172 w191 w203 w206 w219 w233 w241 w271 w281 w290 w303 w314 w323 w330 w345 w359 w369 w374 w389 w410 w446 w470 w488 w501 w513 w518 w537]
              tunnel: [w55 w60 w85 w91 w106 w121 w127 w136 w145 w152 w162 w172 w191 w203 w206 w219 w233 w240 w271 w281 w287 w301 w314 w323 w329 w344 w359 w369 w373 w388 w410 w446 w470 w488 w501 w513 w518 w537] -> w44
              frame "Start" {
                n15 = call "Initialise Devices API.vi"("Error In"=w57) -> ("Error Out"=w56:errorcluster)  [unwired: 10 in]
              }
              frame "Initialise Devices" {
                n16 = Unbundle By Name(w65) -> ("Colour wheel"=w73:T29, "File IO"=w70:T30, "Scope"=w77:T18, "Monochromator"=w68:T9, "DAQ"=w76:T3, "Shutter"=w67:T7)
                n17 = call "Start API.vi"("Shutter"=w67, "Error In"=w64) -> ("Error Out"=w74:errorcluster)  [unwired: 9 in]
                n18 = call "Calculate parameters API.vi"("DAQ"=w76, "Error In"=w74) -> ("Error Out"=w75:errorcluster)  [unwired: 9 in]
                n19 = call "Start API.vi"("Error In"=w75) -> ("Error Out"=w66:errorcluster)  [unwired: 10 in]
                n20 = call "Start API.vi"("Monochromator"=w68, "Error In"=w66) -> ("Error Out"=w69:errorcluster)  [unwired: 9 in]
                n21 = call "Calculate parameters API.vi"("Scope"=w77, "Error In"=w69) -> ("Error Out"=w78:errorcluster)  [unwired: 9 in]
                n22 = call "Start API.vi"("Error In"=w78) -> ("Error Out"=w79:errorcluster)  [unwired: 10 in]
                n23 = call "Start API.vi"("File IO parameters"=w70, "Error In"=w79) -> ("Error Out"=w71:errorcluster)  [unwired: 9 in]
                n24 = call "Start API.vi"("Colour wheel"=w73, "Error In"=w71) -> ("Error Out"=w72:errorcluster)  [unwired: 9 in]
                n25 = call "Start API.vi"("Config"=w65, "Error In"=w72) -> ("Error Out"=w63:errorcluster)  [unwired: 9 in]
                n26 = case shown="True" w61 {
                  tunnel: w63 -> [w80 w82]
                  tunnel: [w80 w81] -> w62
                  frame False {
                  }
                  frame True {
                    n27 = call "Set Spectrum Setup API.vi"("Error In"=w82) -> ("Error Out"=w81:errorcluster)  [unwired: 10 in]
                  }
                }
              }
              frame "End Test" {
                n28 = Bundle By Name(cluster=w86, "Test Complete"=TRUE) -> (w85:T31)
              }
              frame "Stop" {
                n29 = call "Stop API.vi"("Error In"=w98) -> ("Error Out"=w100:errorcluster)  [unwired: 10 in]
                n30 = call "Stop API.vi"("Error In"=w100) -> ("Error Out"=w99:errorcluster)  [unwired: 10 in]
                n31 = call "Stop API.vi"("Error In"=w99) -> ("Error Out"=w96:errorcluster)  [unwired: 10 in]
                n32 = call "Stop API.vi"("Error In"=w96) -> ("Error Out"=w95:errorcluster)  [unwired: 10 in]
                n33 = call "Stop API.vi"("Error In"=w95) -> ("Error Out"=w94:errorcluster)  [unwired: 10 in]
                n34 = call "Stop API.vi"("Error In"=w94) -> ("Error Out"=w93:errorcluster)  [unwired: 10 in]
                n35 = call "Stop API.vi"("Error In"=w93) -> ("Error Out"=w90:errorcluster)  [unwired: 10 in]
                n36 = Flush Event Queue(3:w90) -> (11:w89:errorcluster)  [unwired: 5 in, 2 out]
              }
              frame "Set DAQ data" {
                n37 = Variant To Data(error in=w113, type=T3 {"Data"={"Live"={"t0"=timestamp(0 s since 1904-01-01), "dt"=1.0, "Y"=[]}, "Accumulated"={"t0"=timestamp(0 s since 1904-01-01), "dt"=1.0, "Y"=[]}, "Averaged"={"t0"=timestamp(0 s since 1904-01-01), "dt"=1.0, "Y"=[]}, "data array"=[], "live time array"=[], "Live (decimated)"={"t0"=timestamp(0 s since 1904-01-01), "dt"=1.0, "Y"=[]}}, "Config"={"Input Config"=0, "Card"=enum."USB-6211", "100% Reflectance Standard (V)"=0.0, "Input Channel"="Dev1/ai0", "Average number of points"=0.0, "Trigger Level (V)"=0.0, "Rate (Hz)"=0, "End Time (s)"=0.0}, "Indicators"={"Final number of points"=0.0, "Number of samples"=0.0, "dt"=0.0, "Shots"=10, "Shot counter"=10, "Test counter"=10, "Background level (V)"=0.0, "DAQ task"="", "timestamp of data"=timestamp(0 s since 1904-01-01), "Test Type"=enum."A-Test"}} ("DAQ"), Variant=w112) -> (data=w110:T3, error out=w108:errorcluster)
                n38 = Bundle By Name(cluster=w109, "DAQ"=w110) -> (w104:T2)
                n39 = Unbundle By Name(w104) -> ("Test.Config.Amplification Factor"=w105:dbl, "DAQ.Indicators.Background level (V)"=w102:dbl)
                n40 = Multiply(x=w105, y=w102) -> (x*y=w101:dbl)
                n41 = Bundle By Name(cluster=w104, "Test.Indicators.Scope Background Level (Amps)"=w101, "Test.Indicators.DAQ Background Level (V)"=w102) -> (w103:T2)
              }
              frame "Set Scope data" {
                # "Updates the main controller's scope config"
                n42 = Variant To Data(error in=w126, type=T18 {"Config"={"VISA Resource"="COM1", "Model"=enum."DPO 2012B", "Timebase"=0.2, "Timeout (ms)"=0, "TAS"={"Vertical Range (V)"=0.0, "Vertical Offset (0.0 divs)"=0.0, "Bandwidth"=0, "Probe Attenuation (10.0)"=0.0, "Vertical Coupling"=1, "Impedance"=2, "Multiplication factor"=1.0, "Channel"=enum."Channel 1"}, "TPC"={"Vertical Range (V)"=0.2, "Vertical Offset (0.0 divs)"=0.0, "Bandwidth"=0, "Probe Attenuation (10.0)"=0.0, "Vertical Coupling"=1, "Impedance"=1, "Multiplication factor"=2.0, "Channel"=enum."B1"}, "Trigger"={"Mode"=enum."Laser (TAS)", "Source "=enum."Channel 1", "PIA"={"Test LEDs"=FALSE, "LED line"="", "LED off (s)"=0.0, "LED on (s)"=0.0}, "Threshold (V)"=10000.0}}, "Indicators"={"Setup"={"Final number of points"=10000.0, "Pretrigger points"=1000.0, "Number of readouts"=0, "Model"={"Acquisition Type"=2, "Record length (points)"=10, "Averages on scope"=1, "Average number of points"=10000.0}}, "Timestamp of Data"=timestamp(0 s since 1904-01-01)}, "Data"={"TPC"={"Live data"={"t0"=timestamp(0 s since 1904-01-01), "dt"=1.0, "Y"=[]}, "Averaged data"={"t0"=timestamp(0 s since 1904-01-01), "dt"=1.0, "Y"=[]}, "Accumulated data"={"t0"=timestamp(0 s since 1904-01-01), "dt"=1.0, "Y"=[]}, "Final data"={"t0"=timestamp(0 s since 1904-01-01), "dt"=1.0, "Y"=[]}}, "TAS"={"Live data"={"t0"=timestamp(0 s since 1904-01-01), "dt"=1.0, "Y"=[]}, "Averaged data"={"t0"=timestamp(0 s since 1904-01-01), "dt"=1.0, "Y"=[]}, "Accumulated data"={"t0"=timestamp(0 s since 1904-01-01), "dt"=1.0, "Y"=[]}, "Final data"={"t0"=timestamp(0 s since 1904-01-01), "dt"=1.0, "Y"=[]}}, "Time arrays"={"Time array (decimated)"=[], "waveform"={"t0"=timestamp(0 s since 1904-01-01), "dt"=1.0, "Y"=[]}}}, "Test"={"Config"={"Amplification Factor"=2.0, "100% Reflectance Standard"=2.0, "Calculation Method"=enum."Reflectance", "Option to discard new data?"=FALSE, "Mode"=enum."Spectrum", "Number of Averages"=0, "B Test?"=FALSE}, "Indicators"={"DAQ Background Level (V)"=2.0, "A-Test Counter"=2, "B-Test Counter"=2, "Type"=enum."A-Test", "Scope Background Level (Amps)"=2.0, "TAS only?"=FALSE}}} ("Scope"), Variant=w125) -> (data=w118:T18, error out=w120:errorcluster)
                n43 = Unbundle By Name(w118) -> ("Test.Indicators.A-Test Counter"=w115:i32, "Test.Indicators.B-Test Counter"=w114:i32)
                n44 = Bundle By Name(cluster=w124, "Scope"=w118, "Test.Indicators.A-Test Counter"=w115, "Test.Indicators.B-Test Counter"=w114) -> (w117:T2)
                n45 = Unbundle By Name(w117) -> ("Test"=w116:T15)
                n46 = call "Update Test Info API.vi"("Error In"=w120, "Test"=w116) -> ("Error Out"=w119:errorcluster)  [unwired: 9 in]
              }
              frame "Set Monochromator data" {
                n47 = Variant To Data(error in=w135, type=T9 {"Type"=enum."PTI", "Wavelength (nm)"=600.0, "Grating, gr/mm"=enum."1200", "Grating mode"=enum."Unknown", "Spectrum mode"={"Spectrum mode?"=FALSE, "Start wavelength (nm)"=0.0, "End wavelength (nm)"=0.0, "Wavelength step (nm)"=0.0, "Wavelength array"=[], "array index"=0}, "PTI"={"Delay before read (ms)"=50, "Mono 1"={"Timeout (ms)"=1000, "Resource Name"="COM1", "Baud Rate"=9600, "Data Bits"=8, "Parity"=0, "Stop Bits"=10, "Flow Control"=0}, "Mono 2"={"Timeout (ms)"=1000, "Resource Name"="COM1", "Baud Rate"=9600, "Data Bits"=8, "Parity"=0, "Stop Bits"=10, "Flow Control"=0}, "Two PTI Monochromators?"=FALSE}, "Oriel (custom)"={"reference"=refnum}, "Force wavelength confirmation (PTI)?"=FALSE} ("Monochromator"), Variant=w134) -> (data=w133:T9, error out=w129:errorcluster)
                n48 = Bundle By Name(cluster=w132, "Monochromator"=w133) -> (w131:T2)
              }
              frame "Set colour wheel data" {
                n49 = Variant To Data(error in=w144, type=T29 {"Reference"=600, "Colour Wheel Wavelengths"=[], "Waveform Index"=0, "COM Port"="", "Enabled?"=FALSE} ("Colour wheel"), Variant=w143) -> (data=w142:T29, error out=w138:errorcluster)
                n50 = Bundle By Name(cluster=w141, "Colour wheel"=w142) -> (w140:T2)
              }
              frame "Set all config data" {
                n51 = Variant To Data(error in=w151, type=w147, Variant=w150) -> (data=w148:T2, error out=w149:errorcluster)
              }
              frame "Set Spectrum Setup" {
                n52 = Unbundle By Name(w153) -> ("Test.Config.Mode"=w156:enum32{"Spectrum", "Kinetic"})
                n53 = case shown="\"Kinetic\"" w156 {
                  tunnel: [w158 w160] -> w154
                  tunnel: w155 -> [w159 w161]
                  frame "Spectrum" {
                    # "Generates an array of wavelengths"
                    n54 = call "Spectrum Setup API.vi"("Error In"=w159) -> ("Error Out"=w158:errorcluster)  [unwired: 10 in]
                  }
                  frame "Kinetic" {
                    n55 = call "Spectrum Setup Complete API.vi"("Error In"=w161) -> ("Error Out"=w160:errorcluster)  [unwired: 10 in]
                  }
                }
              }
              frame "Spectrum Setup Complete" {
                n56 = case shown="True" w163 {
                  tunnel: w165 -> [w167 w169]
                  tunnel: [w167 w168] -> w164
                  frame False {
                  }
                  frame True {
                    n57 = call "Set Monochromator Setup API.vi"("Error In"=w169) -> ("Error Out"=w168:errorcluster)  [unwired: 10 in]
                  }
                }
              }
              frame "Set Monochromator Setup" {
                n58 = Unbundle By Name(w170) -> ("Test.Config.Mode"=w175:enum32{"Spectrum", "Kinetic"}, "Monochromator.Wavelength (nm)"=w174:dbl)
                n59 = case shown="\"Spectrum\"" w175 {
                  tunnel: [w178 w180] -> w173
                  tunnel: w171 -> [w177 w181]
                  tunnel: w174 -> [_ w179]
                  frame "Spectrum" {
                    # "Moves monochromator to the first wavelength in the spectrum array"
                    n60 = call "Spectrum Move API.vi"("Error In"=w177) -> ("Error Out"=w178:errorcluster)  [unwired: 10 in]
                  }
                  frame "Kinetic" {
                    # "Moves monochromator to setup wavelength"
                    n61 = call "Monochromator Setup API.vi"("Error In"=w181, "wavelength"=w179) -> ("Error Out"=w180:errorcluster)  [unwired: 9 in]
                  }
                }
              }
              frame "Monochromator Setup Complete" {
                n62 = Unbundle By Name(w187) -> ("Monochromator.Wavelength (nm)"=w188:dbl)
                n63 = Format Into String(format string="%#g", w188) -> (resulting string=w183:string)  [unwired: 2 in, 1 out]
                n64 = Concatenate Strings(w183, "nm" ("string")) -> (w182:string)
                n65 = Bundle By Name(cluster=w187, "File IO.File prefix"=w182) -> (w186:T2)
                n66 = call "Update File Prefix API.vi"("Error In"=w189, "File Prefix"=w182) -> ("Error Out"=w190:errorcluster)  [unwired: 9 in]
                n67 = case shown="True" w192 {
                  tunnel: w190 -> [w194 w196]
                  tunnel: [w194 w195] -> w193
                  frame False {
                  }
                  frame True {
                    n68 = call "Set Colour Wheel Setup API.vi"("Error In"=w196) -> ("Error Out"=w195:errorcluster)  [unwired: 10 in]
                  }
                }
              }
              frame "Set Colour Wheel Setup" {
                # "The colour wheel requires the monochromator to spit out its current wavelength before it can move to that wavelength"
                n69 = Unbundle By Name(w198) -> ("Monochromator.Wavelength (nm)"=w200:dbl, "Colour wheel.Colour Wheel Wavelengths"=w197:dbl[])
                n70 = call "Monochromator Wavelength to Colour Wheel Enum.vi"("error in (no error)"=w202, "Possible Wavelengths"=w197, "Wavelength (nm)"=w200) -> ("error out"=w201:errorcluster, "Index"=w199:i32)  [unwired: 7 in]
                n71 = call "Move API.vi"("Error In"=w201, "Index"=w199) -> ("Error Out"=w204:errorcluster)  [unwired: 9 in]
              }
              frame "Colour Wheel Setup Complete" {
                n72 = case shown="True" w207 {
                  tunnel: w209 -> [w211 w213]
                  tunnel: [w211 w212] -> w208
                  frame False {
                  }
                  frame True {
                    n73 = call "Move Shutter API.vi"("Error In"=w213) -> ("Error Out"=w212:errorcluster)  [unwired: 10 in]
                  }
                }
              }
              frame "Move Shutter" {
                n74 = Unbundle By Name(w217) -> ("Test.Config.Mode"=w214:enum32{"Spectrum", "Kinetic"}, "Test.Indicators.Type"=w218:T6)
                n75 = case shown="\"A-Test\"" w218 {
                  tunnel: w215 -> [w224 w230]
                  tunnel: [w221 w229] -> w216
                  tunnel: w214 -> [w223 _]
                  frame "A-Test" {
                    n76 = call "Move Shutter Complete API.vi"("Error In"=w224) -> ("Error Out"=w222:errorcluster)  [unwired: 10 in]
                    n77 = case shown="\"Spectrum\"" w223 {
                      tunnel: w222 -> [w226 w227]
                      tunnel: [w226 w227] -> w221
                      frame "Spectrum" {
                        n78 = Wait (ms)(milliseconds to wait=u32 20000) -> ()  [unwired: 1 out]
                      }
                      frame "Kinetic" {
                      }
                    }
                  }
                  frame "B-Test" {
                    w228 = u32 10000  # Wait (ms)
                    n79 = call "Move API.vi"("Error In"=w230, "Wait (ms)"=w228) -> ("Error Out"=w229:errorcluster)  [unwired: 9 in]
                  }
                }
              }
              frame "Move Shutter Complete" {
                n80 = case shown="True" w234 {
                  tunnel: w235 -> [w236 w238]
                  tunnel: [w236 w237] -> w231
                  frame False {
                  }
                  frame True {
                    n81 = call "Collect Data API.vi"("Error In"=w238) -> ("Error Out"=w237:errorcluster)  [unwired: 10 in]
                  }
                }
              }
              frame "Collect Data" {
                # "#MP Check whether to stop A Test or B Test here"
                # "#MP Check for B-test is now done in \n'All Finalising Complete' case."
                n82 = Unbundle By Name(w245) -> ("Test"=w249:T15, "Test.Indicators.Type"=w239:T6)
                n83 = case shown="\"A-Test\"" w239 {
                  tunnel: w249 -> [w252 w256]
                  tunnel: [w251 w255] -> w244
                  frame "A-Test" {
                    n84 = Unbundle By Name(w252) -> ("Config.Number of Averages"=w253:i32)
                    n85 = call "GetTestCounter.vi"("Test"=w252) -> ("Current test counter"=w254:i32)  [unwired: 10 in]
                    n86 = Greater Or Equal?(x=w254, y=w253) -> (x >= y?=w251:bool)
                  }
                  frame "B-Test" {
                    n87 = call "GetTestCounter.vi"("Test"=w256) -> ("Current test counter"=w258:i32)  [unwired: 10 in]
                    n88 = Unbundle By Name(w256) -> ("Indicators.A-Test Counter"=w257:i32)
                    n89 = Greater Or Equal?(x=w258, y=w257) -> (x >= y?=w255:bool)
                  }
                }
                n90 = Unbundle By Name(w241) -> ("Test Complete"=w242:bool)
                n91 = Or(x=w242, y=w244) -> (x .or. y?=w243:bool)
                n92 = case shown="False" w243 {
                  tunnel: [w260 w267] -> w246
                  tunnel: w245 -> [w260 w267]
                  tunnel: [w261 w268] -> w247
                  tunnel: w248 -> [w262 w269]
                  tunnel: w241 -> [w259 w266]
                  tunnel: [w259 w264] -> w240
                  frame False {
                    # "Continue to get and accumulate data"
                    n93 = call "Acquire DAQ and scope data API.vi"("Error In"=w262) -> ("Error Out"=w263:errorcluster)  [unwired: 10 in]
                    n94 = call "Accumulate test data API.vi"("Error In"=w263) -> ("Error Out"=w261:errorcluster)  [unwired: 10 in]
                  }
                  frame True {
                    # "End of test data acquisition. Time to average, finalise, and process data"
                    n95 = call "Collect Data Complete API.vi"("Error In"=w269) -> ("Error Out"=w268:errorcluster)  [unwired: 10 in]
                    n96 = Bundle By Name(cluster=w266, "Test Complete"=FALSE ("DAQ Acq Complete")) -> (w264:T31)
                  }
                }
              }
              frame "Acquire test data" {
                n97 = Unbundle By Name(w270) -> ("Scope.Indicators.Setup.Model.Averages on scope"=w273:i32)
                n98 = call "Start acquisition API.vi"("Error In"=w274) -> ("Error Out"=w278:errorcluster)  [unwired: 10 in]
                n99 = call "Get test data API.vi"("Error In"=w278) -> ("Error Out"=w277:errorcluster)  [unwired: 10 in]
                n100 = call "Get test data API.vi"("Error In"=w274, "Shots"=w273) -> ("Error Out"=w276:errorcluster)  [unwired: 9 in]
                n101 = Merge Errors(w277, w276) -> (w275:errorcluster)
              }
              frame "Accumulate test data" {
                n102 = call "Accumulate data API.vi"("Error In"=w279) -> ("Error Out"=w284:errorcluster)  [unwired: 10 in]
                n103 = call "Accumulate data API.vi"("Error In"=w279) -> ("Error Out"=w285:errorcluster)  [unwired: 10 in]
                n104 = Merge Errors(w285, w284) -> (w283:errorcluster)
              }
              frame "DAQ Acquisition Complete" {
                n105 = Bundle By Name(cluster=w290, "DAQ Acq Complete"=TRUE) -> (w286:T31)
                n106 = Unbundle By Name(w286) -> ("DAQ Acq Complete"=w291:bool, "Scope Acq Complete"=w288:bool)
                n107 = And(x=w291, y=w288) -> (x .and. y?=w292:bool)
                n108 = case shown="True" w292 {
                  tunnel: [w296 w298] -> w287
                  tunnel: w286 -> [w296 w299]
                  frame False {
                  }
                  frame True {
                    w297 = FALSE ("DAQ Acq Complete")
                    n109 = Bundle By Name(cluster=w299, "DAQ Acq Complete"=w297, "Scope Acq Complete"=w297) -> (w298:T31)
                    n110 = call "Collect Data API.vi"() -> ()  [unwired: 11 in, 1 out]
                  }
                }
              }
              frame "Scope Acquisition Complete" {
                n111 = Bundle By Name(cluster=w303, "Scope Acq Complete"=TRUE ("DAQ Acq Complete")) -> (w302:T31)
                n112 = Unbundle By Name(w302) -> ("DAQ Acq Complete"=w306:bool, "Scope Acq Complete"=w304:bool)
                n113 = And(x=w306, y=w304) -> (x .and. y?=w300:bool)
                n114 = case shown="False" w300 {
                  tunnel: [w310 w312] -> w301
                  tunnel: w302 -> [w310 w313]
                  frame False {
                  }
                  frame True {
                    w311 = FALSE ("Scope Acq Complete")
                    n115 = Bundle By Name(cluster=w313, "DAQ Acq Complete"=w311, "Scope Acq Complete"=w311) -> (w312:T31)
                    n116 = call "Collect Data API.vi"() -> ()  [unwired: 11 in, 1 out]
                  }
                }
              }
              frame "Collect Data Complete" {
                n117 = case shown="True" w315 {
                  tunnel: w317 -> [w319 w321]
                  tunnel: [w319 w320] -> w316
                  frame False {
                  }
                  frame True {
                    n118 = call "Average test data API.vi"("Error In"=w321) -> ("Error Out"=w320:errorcluster)  [unwired: 10 in]
                  }
                }
              }
              frame "Average test data" {
                n119 = call "Average data API.vi"("Error In"=w328) -> ("Error Out"=w326:errorcluster)  [unwired: 10 in]
                n120 = call "Average data API.vi"("Error In"=w328) -> ("Error Out"=w327:errorcluster)  [unwired: 10 in]
                n121 = Merge Errors(w327, w326) -> (w325:errorcluster)
              }
              frame "DAQ Averaging Complete" {
                n122 = Bundle By Name(cluster=w330, "DAQ Average Complete"=TRUE ("DAQ Acq Complete")) -> (w332:T31)
                n123 = Unbundle By Name(w332) -> ("DAQ Average Complete"=w335:bool, "Scope Average Complete"=w333:bool)
                n124 = And(x=w335, y=w333) -> (x .and. y?=w331:bool)
                n125 = case shown="True" w331 {
                  tunnel: [w339 w340] -> w329
                  tunnel: w332 -> [w339 w341]
                  frame False {
                  }
                  frame True {
                    w342 = FALSE ("Scope Average Complete")
                    n126 = Bundle By Name(cluster=w341, "Scope Average Complete"=w342, "DAQ Average Complete"=w342) -> (w340:T31)
                    n127 = call "All Averaging Complete API.vi"() -> ()  [unwired: 11 in, 1 out]
                  }
                }
              }
              frame "Scope Averaging Complete" {
                n128 = Bundle By Name(cluster=w345, "Scope Average Complete"=TRUE ("DAQ Acq Complete")) -> (w346:T31)
                n129 = Unbundle By Name(w346) -> ("DAQ Average Complete"=w349:bool, "Scope Average Complete"=w347:bool)
                n130 = And(x=w349, y=w347) -> (x .and. y?=w343:bool)
                n131 = case shown="False" w343 {
                  tunnel: [w353 w355] -> w344
                  tunnel: w346 -> [w353 w356]
                  frame False {
                  }
                  frame True {
                    w354 = FALSE ("Scope Finalising Complete")
                    n132 = Bundle By Name(cluster=w356, "DAQ Average Complete"=w354, "DAQ Average Complete"=w354) -> (w355:T31)
                    n133 = call "All Averaging Complete API.vi"() -> ()  [unwired: 11 in, 1 out]
                  }
                }
              }
              frame "All Averaging Complete" {
                n134 = call "Finalise test data API.vi"("Error In"=w358) -> ("Error Out"=w357:errorcluster)  [unwired: 10 in]
              }
              frame "Finalise test data" {
                n135 = call "Average Pre Trigger Data API.vi"("Error In"=w365) -> ("Error Out"=w364:errorcluster)  [unwired: 10 in]
                n136 = call "Background voltage API.vi"("Error In"=w364) -> ("Error Out"=w363:errorcluster)  [unwired: 10 in]
                n137 = flat-sequence {
                  tunnel: w363 -> [w371]
                  tunnel: [w371] -> w362
                  frame #0 {
                    n138 = Wait (ms)(milliseconds to wait=u32 200) -> ()  [unwired: 1 out]
                  }
                }
                n139 = call "Add background voltage API.vi"("Error In"=w362) -> ("Error Out"=w368:errorcluster)  [unwired: 10 in]
                n140 = call "Scale TPC API.vi"("Error In"=w368) -> ("Error Out"=w366:errorcluster)  [unwired: 10 in]
              }
              frame "DAQ Finalising Complete" {
                n141 = Bundle By Name(cluster=w374, "DAQ Finalising Complete"=TRUE ("DAQ Acq Complete")) -> (w376:T31)
                n142 = Unbundle By Name(w376) -> ("DAQ Finalising Complete"=w379:bool, "Scope Finalising Complete"=w377:bool)
                n143 = And(x=w379, y=w377) -> (x .and. y?=w375:bool)
                n144 = case shown="False" w375 {
                  tunnel: [w383 w384] -> w373
                  tunnel: w376 -> [w383 w385]
                  frame False {
                  }
                  frame True {
                    w386 = FALSE ("Scope Average Complete")
                    n145 = Bundle By Name(cluster=w385, "DAQ Finalising Complete"=w386, "Scope Finalising Complete"=w386) -> (w384:T31)
                    n146 = call "All Finalise Complete API.vi"() -> ()  [unwired: 11 in, 1 out]
                  }
                }
              }
              frame "Scope Finalising Complete" {
                n147 = Bundle By Name(cluster=w389, "Scope Finalising Complete"=TRUE ("DAQ Acq Complete")) -> (w390:T31)
                n148 = Unbundle By Name(w390) -> ("DAQ Finalising Complete"=w393:bool, "Scope Finalising Complete"=w391:bool)
                n149 = And(x=w393, y=w391) -> (x .and. y?=w387:bool)
                n150 = case shown="True" w387 {
                  tunnel: [w397 w399] -> w388
                  tunnel: w390 -> [w397 w400]
                  frame False {
                  }
                  frame True {
                    w398 = FALSE ("Scope Finalising Complete")
                    n151 = Bundle By Name(cluster=w400, "DAQ Finalising Complete"=w398, "Scope Finalising Complete"=w398) -> (w399:T31)
                    n152 = call "All Finalise Complete API.vi"() -> ()  [unwired: 11 in, 1 out]
                  }
                }
              }
              frame "All Finalising Complete" {
                n153 = Unbundle By Name(w409) -> ("Test.Config.B Test?"=w402:bool, "Test.Indicators.Type"=w405:T6)
                n154 = Equal?(x=w405, y=Test_Type."A-Test" ("Test.Indicators.Type")) -> (x = y?=w403:bool)
                n155 = And(x=w402, y=w403) -> (x .and. y?=w401:bool)
                n156 = case shown="True" w401 {
                  tunnel: w407 -> [w414 w417]
                  tunnel: [w415 w432] -> w404
                  tunnel: w409 -> [w412 w430]
                  tunnel: [w412 w431] -> w408
                  frame False {
                    # "If the current test is B-Test or the user has selected not to run a B test we carry on to the post-processing steps."
                    n157 = call "Save parameters API.vi"("Error In"=w414, "Config"=w412) -> ("Error Out"=w413:errorcluster)  [unwired: 9 in]
                    n158 = call "Process test data API.vi"("Error In"=w413) -> ("Error Out"=w415:errorcluster)  [unwired: 10 in]
                  }
                  frame True {
                    w419 = 0 ("DAQ.Indicators.Shot counter")
                    w425 = Test_Type."B-Test" ("Test.Indicators.Type")
                    # "If the current test is A-Test we want to repeat it but as a B-Test"
                    n159 = Bundle By Name(cluster=w430, "Test.Indicators.Type"=w425, "Scope.Test.Indicators.Type"=w425, "DAQ.Indicators.Test Type"=w425, "DAQ.Indicators.Shot counter"=w419, "DAQ.Indicators.Test counter"=w419, "DAQ.Data"=T35 {"Live"={"t0"=timestamp(0 s since 1904-01-01), "dt"=1.0, "Y"=[]}, "Accumulated"={"t0"=timestamp(0 s since 1904-01-01), "dt"=1.0, "Y"=[]}, "Averaged"={"t0"=timestamp(0 s since 1904-01-01), "dt"=1.0, "Y"=[]}, "data array"=[], "live time array"=[], "Live (decimated)"={"t0"=timestamp(0 s since 1904-01-01), "dt"=1.0, "Y"=[]}} ("Data"), "Scope.Data"=T27 {"TPC"={"Live data"={"t0"=timestamp(0 s since 1904-01-01), "dt"=1.0, "Y"=[]}, "Averaged data"={"t0"=timestamp(0 s since 1904-01-01), "dt"=1.0, "Y"=[]}, "Accumulated data"={"t0"=timestamp(0 s since 1904-01-01), "dt"=1.0, "Y"=[]}, "Final data"={"t0"=timestamp(0 s since 1904-01-01), "dt"=1.0, "Y"=[]}}, "TAS"={"Live data"={"t0"=timestamp(0 s since 1904-01-01), "dt"=1.0, "Y"=[]}, "Averaged data"={"t0"=timestamp(0 s since 1904-01-01), "dt"=1.0, "Y"=[]}, "Accumulated data"={"t0"=timestamp(0 s since 1904-01-01), "dt"=1.0, "Y"=[]}, "Final data"={"t0"=timestamp(0 s since 1904-01-01), "dt"=1.0, "Y"=[]}}, "Time arrays"={"Time array (decimated)"=[], "waveform"={"t0"=timestamp(0 s since 1904-01-01), "dt"=1.0, "Y"=[]}}} ("Data")) -> (w431:T2)
                    n160 = call "Clear Graphs API.vi"("Error In"=w417) -> ("Error Out"=w416:errorcluster)  [unwired: 10 in]
                    n161 = Unbundle By Name(w431) -> ("DAQ"=w420:T3, "Scope"=w427:T18)
                    n162 = call "Stop API.vi"("Error In"=w416) -> ("Error Out"=w429:errorcluster)  [unwired: 10 in]
                    n163 = call "Calculate parameters API.vi"("Scope"=w427, "Error In"=w429) -> ("Error Out"=w428:errorcluster)  [unwired: 9 in]
                    n164 = call "Start API.vi"("Error In"=w428) -> ("Error Out"=w422:errorcluster)  [unwired: 10 in]
                    n165 = call "Stop API.vi"("Error In"=w422) -> ("Error Out"=w423:errorcluster)  [unwired: 10 in]
                    n166 = call "Calculate parameters API.vi"("DAQ"=w420, "Error In"=w423) -> ("Error Out"=w424:errorcluster)  [unwired: 9 in]
                    n167 = call "Start API.vi"("Error In"=w424) -> ("Error Out"=w421:errorcluster)  [unwired: 10 in]
                    n168 = call "Move Shutter API.vi"("Error In"=w421) -> ("Error Out"=w432:errorcluster)  [unwired: 10 in]
                  }
                }
              }
              frame "Process test data" {
                w439 = "A-Test DAQ (raw data)" ("DAQ average file")
                w440 = "A-Test Scope TAS (No BG)" ("DAQ average file")
                # "Read the DAQ text file and process it (creates a new \"final\" file)"
                # "Read the scope text file and process it (creates a new \"final\" file)"
                n169 = flat-sequence {
                  tunnel: w434 -> [w449]
                  tunnel: [w449] -> w433
                  frame #0 {
                    n170 = Wait (ms)(milliseconds to wait=u32 3000) -> ()  [unwired: 1 out]
                  }
                }
                n171 = call "Read waveform API.vi"("Error In"=w433, "Waveform name"=w439) -> ("Error Out"=w443:errorcluster)  [unwired: 9 in]
                n172 = call "Send waveform API.vi"("Error In"=w443, "Waveform name"=w439) -> ("Error Out"=w448:errorcluster)  [unwired: 9 in]
                n173 = call "Read waveform API.vi"("Error In"=w448, "Waveform name"=w440) -> ("Error Out"=w447:errorcluster)  [unwired: 9 in]
                n174 = call "Send waveform API.vi"("Error In"=w447, "Waveform name"=w440) -> ("Error Out"=w442:errorcluster)  [unwired: 9 in]
                n175 = Unbundle By Name(w436) -> ("Test.Config.B Test?"=w435:bool)
                n176 = call "Delete waveform API.vi"("Error In"=w442, "Waveform name"=w440) -> ("Error Out"=w441:errorcluster)  [unwired: 9 in]
                n177 = case shown="True" w435 {
                  tunnel: w441 -> [w451 w453]
                  tunnel: [w451 w457] -> w438
                  frame False {
                  }
                  frame True {
                    w456 = "B-Test DAQ (raw data)" ("DAQ average file")
                    w458 = "B-Test Scope TAS (No BG)" ("DAQ average file")
                    n178 = flat-sequence {
                      tunnel: w453 -> [w461]
                      tunnel: [w461] -> w452
                      frame #0 {
                        n179 = Wait (ms)(milliseconds to wait=u32 3000) -> ()  [unwired: 1 out]
                      }
                    }
                    n180 = call "Read waveform API.vi"("Error In"=w452, "Waveform name"=w456) -> ("Error Out"=w455:errorcluster)  [unwired: 9 in]
                    n181 = call "Send waveform API.vi"("Error In"=w455, "Waveform name"=w456) -> ("Error Out"=w454:errorcluster)  [unwired: 9 in]
                    n182 = call "Read waveform API.vi"("Error In"=w454, "Waveform name"=w458) -> ("Error Out"=w460:errorcluster)  [unwired: 9 in]
                    n183 = call "Send waveform API.vi"("Error In"=w460, "Waveform name"=w458) -> ("Error Out"=w459:errorcluster)  [unwired: 9 in]
                    n184 = call "Delete waveform API.vi"("Error In"=w459, "Waveform name"=w458) -> ("Error Out"=w457:errorcluster)  [unwired: 9 in]
                  }
                }
                n185 = flat-sequence {
                  tunnel: w438 -> [w463]
                  tunnel: [w463] -> w437
                  frame #0 {
                    n186 = Wait (ms)(milliseconds to wait=u32 2000) -> ()  [unwired: 1 out]
                  }
                }
                n187 = call "A-B Processing API.vi"("Error In"=w437) -> ("Error Out"=w445:errorcluster)  [unwired: 10 in]
              }
              frame "A-B Processing" {
                n188 = Unbundle By Name(w469) -> ("File IO"=w465:T30, "Test.Config.B Test?"=w466:bool)
                n189 = case shown="True" w466 {
                  tunnel: [w472 w474] -> w468
                  tunnel: w465 -> [_ w478]
                  tunnel: w467 -> [w473 w481]
                  frame False {
                    n190 = call "A-B Processing Complete API.vi"("Error In"=w473) -> ("Error Out"=w472:errorcluster)  [unwired: 10 in]
                  }
                  frame True {
                    n191 = call "Scope A-B Processing API.vi"("Error In"=w481, "Filename (B)"="B-Test Scope TAS (Pre Trigger Averaged)" ("DAQ average file"), "Filename (A)"="A-Test Scope TAS (Pre Trigger Averaged)" ("DAQ average file"), "File IO"=w478) -> ("Error Out"=w480:errorcluster)  [unwired: 7 in]
                    n192 = flat-sequence {
                      tunnel: w480 -> [w486]
                      tunnel: [w486] -> w479
                      frame #0 {
                        n193 = Wait (ms)(milliseconds to wait=u32 2000) -> ()  [unwired: 1 out]
                      }
                    }
                    n194 = call "DAQ A-B Processing API.vi"("Error In"=w479, "Filename (B)"="B-Test DAQ (raw data)" ("DAQ average file"), "Filename (A)"="A-Test DAQ (raw data)" ("DAQ average file"), "File IO"=w478) -> ("Error Out"=w475:errorcluster)  [unwired: 7 in]
                    n195 = flat-sequence {
                      tunnel: w475 -> [w484]
                      tunnel: [w484] -> w474
                      frame #0 {
                        n196 = Wait (ms)(milliseconds to wait=u32 2000) -> ()  [unwired: 1 out]
                      }
                    }
                  }
                }
              }
              frame "A-B Processing Complete" {
                n197 = case shown="True" w489 {
                  tunnel: w491 -> [w493 w495]
                  tunnel: [w493 w494] -> w490
                  frame False {
                  }
                  frame True {
                    n198 = call "DAQ-Scope Stitching API.vi"("Error In"=w495) -> ("Error Out"=w494:errorcluster)  [unwired: 10 in]
                  }
                }
              }
              frame "DAQ-Scope Stitching" {
                n199 = Unbundle By Name(w498) -> ("Test.Config.B Test?"=w496:bool, "File IO"=w497:T30)
                n200 = case shown="True" w496 {
                  tunnel: w500 -> [w504 w509]
                  tunnel: [w503 w508] -> w499
                  tunnel: w497 -> [_ w507]
                  frame False {
                    n201 = call "DAQ-Scope Stitching Complete API.vi"("Error In"=w504) -> ("Error Out"=w503:errorcluster)  [unwired: 10 in]
                  }
                  frame True {
                    n202 = call "DAQ-Scope Stitching API.vi"("Error In"=w509, "Scope Filename"="Scope TAS (final A-B)" ("Filename (A)"), "DAQ Filename"="A-Test DAQ (final)" ("Filename (A)"), "File IO"=w507) -> ("Error Out"=w508:errorcluster)  [unwired: 7 in]
                  }
                }
              }
              frame "DAQ-Scope Stitching Complete" {
                n203 = case shown="True" w510 {
                  tunnel: w512 -> [w515 w517]
                  tunnel: [w515 w516] -> w511
                  frame False {
                  }
                  frame True {
                    n204 = call "Return Shutter API.vi"("Error In"=w517) -> ("Error Out"=w516:errorcluster)  [unwired: 10 in]
                  }
                }
              }
              frame "Return Shutter" {
                n205 = Unbundle By Name(w519) -> ("Test.Indicators.Type"=w522:T6)
                n206 = case shown="\"B-Test\"" w522 {
                  tunnel: w521 -> [w525 w528]
                  tunnel: [w524 w527] -> w520
                  frame "A-Test" {
                    n207 = call "Return Shutter Complete API.vi"("Error In"=w525) -> ("Error Out"=w524:errorcluster)  [unwired: 10 in]
                  }
                  frame "B-Test" {
                    n208 = call "Return API.vi"("Error In"=w528, "Wait (ms)"=u32 10000) -> ("Error Out"=w527:errorcluster)  [unwired: 9 in]
                  }
                }
              }
              frame "Return Shutter Complete" {
                # "Keeps a track of wavelengths left to move to so we know \nwhen the Spectrum sequence is complete and we can STOP."
                n209 = Unbundle By Name(w530) -> ("Monochromator.Spectrum mode.array index"=w532:u32, "Monochromator.Spectrum mode.Wavelength array"=w533:dbl[], "Test.Config.Mode"=w536:enum32{"Spectrum", "Kinetic"})
                n210 = case shown="\"Spectrum\"" w536 {
                  tunnel: w535 -> [w546 w580]
                  tunnel: [w545 w582] -> w534
                  tunnel: w533 -> [w544 _]
                  tunnel: w532 -> [w543 _]
                  tunnel: [w540 FALSE] -> w531
                  tunnel: w530 -> [w539 w578]
                  tunnel: [w538 w577] -> w529
                  frame "Spectrum" {
                    n211 = Array Size(array=w544) -> (size(s)=w542:i32)
                    n212 = Greater Or Equal?(x=w543, y=w542) -> (x >= y?=w541:bool)
                    n213 = case shown="True" w541 {
                      tunnel: w546 -> [w552 w569]
                      tunnel: [w565 w572] -> w545
                      tunnel: [TRUE FALSE] -> w540
                      tunnel: w539 -> [w554 w570]
                      tunnel: [w553 w570] -> w538
                      frame False {
                        w550 = T17 {"DAQ Background Level (V)"=0.0, "A-Test Counter"=0, "B-Test Counter"=0, "Type"=enum."A-Test", "Scope Background Level (Amps)"=0.0, "TAS only?"=FALSE} ("Test.Indicators")
                        n214 = Bundle By Name(cluster=w554, "Scope.Test.Indicators"=w550, "Test.Indicators"=w550, "DAQ.Indicators.Test Type"=Test_Type."A-Test", "DAQ.Data"=T35 {"Live"={"t0"=timestamp(0 s since 1904-01-01), "dt"=1.0, "Y"=[]}, "Accumulated"={"t0"=timestamp(0 s since 1904-01-01), "dt"=1.0, "Y"=[]}, "Averaged"={"t0"=timestamp(0 s since 1904-01-01), "dt"=1.0, "Y"=[]}, "data array"=[], "live time array"=[], "Live (decimated)"={"t0"=timestamp(0 s since 1904-01-01), "dt"=1.0, "Y"=[]}} ("Data"), "Scope.Data"=T27 {"TPC"={"Live data"={"t0"=timestamp(0 s since 1904-01-01), "dt"=1.0, "Y"=[]}, "Averaged data"={"t0"=timestamp(0 s since 1904-01-01), "dt"=1.0, "Y"=[]}, "Accumulated data"={"t0"=timestamp(0 s since 1904-01-01), "dt"=1.0, "Y"=[]}, "Final data"={"t0"=timestamp(0 s since 1904-01-01), "dt"=1.0, "Y"=[]}}, "TAS"={"Live data"={"t0"=timestamp(0 s since 1904-01-01), "dt"=1.0, "Y"=[]}, "Averaged data"={"t0"=timestamp(0 s since 1904-01-01), "dt"=1.0, "Y"=[]}, "Accumulated data"={"t0"=timestamp(0 s since 1904-01-01), "dt"=1.0, "Y"=[]}, "Final data"={"t0"=timestamp(0 s since 1904-01-01), "dt"=1.0, "Y"=[]}}, "Time arrays"={"Time array (decimated)"=[], "waveform"={"t0"=timestamp(0 s since 1904-01-01), "dt"=1.0, "Y"=[]}}} ("Data")) -> (w553:T2)
                        n215 = call "Clear Graphs API.vi"("Error In"=w552) -> ("Error Out"=w551:errorcluster)  [unwired: 10 in]
                        n216 = Unbundle By Name(w553) -> ("DAQ"=w557:T3, "Scope"=w563:T18)
                        n217 = call "Stop API.vi"("Error In"=w551) -> ("Error Out"=w561:errorcluster)  [unwired: 10 in]
                        n218 = call "Calculate parameters API.vi"("Scope"=w563, "Error In"=w561) -> ("Error Out"=w562:errorcluster)  [unwired: 9 in]
                        n219 = call "Start API.vi"("Error In"=w562) -> ("Error Out"=w559:errorcluster)  [unwired: 10 in]
                        n220 = call "Stop API.vi"("Error In"=w559) -> ("Error Out"=w560:errorcluster)  [unwired: 10 in]
                        n221 = call "Calculate parameters API.vi"("DAQ"=w557, "Error In"=w560) -> ("Error Out"=w558:errorcluster)  [unwired: 9 in]
                        n222 = call "Start API.vi"("Error In"=w558) -> ("Error Out"=w555:errorcluster)  [unwired: 10 in]
                        n223 = flat-sequence {
                          tunnel: w555 -> [w566]
                          tunnel: [w566] -> w556
                          frame #0 {
                            n224 = Wait (ms)(milliseconds to wait=u32 2000) -> ()  [unwired: 1 out]
                          }
                        }
                        n225 = call "Set Monochromator Setup API.vi"("Error In"=w556) -> ("Error Out"=w565:errorcluster)  [unwired: 10 in]
                      }
                      frame True {
                        n226 = flat-sequence {
                          tunnel: w569 -> [w574]
                          tunnel: [w574] -> w568
                          frame #0 {
                            n227 = One Button Dialog(message="Acquisition Complete") -> ()  [unwired: 1 in, 1 out]
                          }
                        }
                        n228 = call "Stop API.vi"("Error In"=w568) -> ("Error Out"=w573:errorcluster)  [unwired: 10 in]
                        n229 = call "Acquisition Complete API.vi"("Error In"=w573) -> ("Error Out"=w572:errorcluster)  [unwired: 10 in]
                      }
                    }
                  }
                  frame "Kinetic" {
                    w576 = T17 {"DAQ Background Level (V)"=0.0, "A-Test Counter"=0, "B-Test Counter"=0, "Type"=enum."A-Test", "Scope Background Level (Amps)"=0.0, "TAS only?"=FALSE} ("Test.Indicators")
                    n230 = Bundle By Name(cluster=w578, "Scope.Test.Indicators"=w576, "Test.Indicators"=w576) -> (w577:T2)
                    n231 = flat-sequence {
                      tunnel: w580 -> [w584]
                      tunnel: [w584] -> w579
                      frame #0 {
                        n232 = One Button Dialog(message="Acquisition Complete") -> ()  [unwired: 1 in, 1 out]
                      }
                    }
                    n233 = call "Stop API.vi"("Error In"=w579) -> ("Error Out"=w583:errorcluster)  [unwired: 10 in]
                    n234 = call "Acquisition Complete API.vi"("Error In"=w583) -> ("Error Out"=w582:errorcluster)  [unwired: 10 in]
                  }
                }
              }
            }
            n235 = call "Update API.vi"("Config"=w50, "Error In"=w46) -> ("Error Out"=w49:errorcluster)  [unwired: 9 in]
          }
          event Value Change {
            n236 = event-data() -> ("NewVal"=w589:T1)  [unwired: 1 in]
            n237 = case shown="\"End Test\"" w589 {
              tunnel: [w592 w594 w596 w598 w601 w605 w609 w611 w614 w617 w619 w621 w623 w625 w627 w629 w630 w631 w632 w633 w634 w635 w636 w637 w638 w639 w640 w641 w642 w643 w644 w645 w646 w647 w648 w649 w650 w651] -> w591
              tunnel: w590 -> [w593 w595 w597 w598 w602 w606 w610 w611 w615 w618 w620 w622 w624 w626 w628 w629 w630 w631 w632 w633 w634 w635 w636 w637 w638 w639 w640 w641 w642 w643 w644 w645 w646 w647 w648 w649 w650 w651]
              tunnel: w588 -> [_ _ _ _ w599 w604 w608 _ w612 w616 _ _ _ _ _ _ _ _ _ _ _ _ _ _ _ _ _ _ _ _ _ _ _ _ _ _ _ _]
              frame "Start" {
                n238 = call "Start API.vi"("Error In"=w593) -> ("Error Out"=w592:errorcluster)  [unwired: 10 in]
              }
              frame "Initialise Devices" {
                n239 = call "Initialise Devices API.vi"("Error In"=w595) -> ("Error Out"=w594:errorcluster)  [unwired: 10 in]
              }
              frame "Stop" {
                n240 = call "Stop API.vi"("Error In"=w597) -> ("Error Out"=w596:errorcluster)  [unwired: 10 in]
              }
              frame "End Test" {
              }
              frame "Set DAQ data" {
                n241 = Unbundle By Name(w599) -> ("DAQ"=w600:T3)
                n242 = call "Set DAQ config API.vi"("DAQ config"=w600, "Error In"=w602) -> ("Error Out"=w601:errorcluster)  [unwired: 9 in]
              }
              frame "Set Scope data" {
                n243 = Unbundle By Name(w604) -> ("Scope"=w603:T18)
                n244 = call "Set scope config API.vi"("Scope"=w603, "Error In"=w606) -> ("Error Out"=w605:errorcluster)  [unwired: 9 in]
              }
              frame "Set Monochromator data" {
                n245 = Unbundle By Name(w608) -> ("Monochromator"=w607:T9)
                n246 = call "Set monochromator data API.vi"("Monochromator"=w607, "Error In"=w610) -> ("Error Out"=w609:errorcluster)  [unwired: 9 in]
              }
              frame "Spectrum Setup Complete" {
              }
              frame "Set colour wheel data" {
                n247 = Unbundle By Name(w612) -> ("Colour wheel"=w613:T29)
                n248 = call "Set colour wheel data API.vi"("Colour wheel"=w613, "Error In"=w615) -> ("Error Out"=w614:errorcluster)  [unwired: 9 in]
              }
              frame "Set all config data" {
                n249 = call "Set all config data API.vi"("Error In"=w618, "Config"=w616) -> ("Error Out"=w617:errorcluster)  [unwired: 8 in, 1 out]
              }
              frame "Acquire test data" {
                n250 = call "Acquire DAQ and scope data API.vi"("Error In"=w620) -> ("Error Out"=w619:errorcluster)  [unwired: 10 in]
              }
              frame "Accumulate test data" {
                n251 = call "Accumulate test data API.vi"("Error In"=w622) -> ("Error Out"=w621:errorcluster)  [unwired: 10 in]
              }
              frame "Average test data" {
                n252 = call "Average test data API.vi"("Error In"=w624) -> ("Error Out"=w623:errorcluster)  [unwired: 10 in]
              }
              frame "Finalise test data" {
                n253 = call "Finalise test data API.vi"("Error In"=w626) -> ("Error Out"=w625:errorcluster)  [unwired: 10 in]
              }
              frame "Process test data" {
                n254 = call "Process test data API.vi"("Error In"=w628) -> ("Error Out"=w627:errorcluster)  [unwired: 10 in]
              }
              frame "Set Spectrum Setup" {
              }
              frame "Set Monochromator Setup" {
              }
              frame "Monochromator Setup Complete" {
              }
              frame "Set Colour Wheel Setup" {
              }
              frame "Colour Wheel Setup Complete" {
              }
              frame "Move Shutter" {
              }
              frame "Move Shutter Complete" {
              }
              frame "Collect Data" {
              }
              frame "Collect Data Complete" {
              }
              frame "A-B Processing" {
              }
              frame "DAQ-Scope Stitching" {
              }
              frame "DAQ-Scope Stitching Complete" {
              }
              frame "A-B Processing Complete" {
              }
              frame "Return Shutter" {
              }
              frame "Return Shutter Complete" {
              }
              frame "DAQ Acquisition Complete" {
              }
              frame "Scope Acquisition Complete" {
              }
              frame "All Averaging Complete" {
              }
              frame "DAQ Averaging Complete" {
              }
              frame "Scope Averaging Complete" {
              }
              frame "All Finalising Complete" {
              }
              frame "DAQ Finalising Complete" {
              }
              frame "Scope Finalising Complete" {
              }
            }
          }
          event User Event {
            n255 = event-data() -> ()  [unwired: 1 in, 5 out]
          }
        }
      }
      frame Error {
        n256 = local read "Standalone"() -> (w659:bool)
        n257 = case shown="False" w659 {
          tunnel: [w664 _] -> w660
          tunnel: w661 -> [w663 w669]
          frame False {
            n258 = case shown="Error" w663 {
              selector: w663 -> [w665 w667]
              tunnel: [w665 w668] -> w664
              frame No Error {
              }
              frame Error {
                n259 = call "Send Error API.vi"("Error Cluster"=w667) -> ("Error Out"=w666:errorcluster)  [unwired: 10 in]
                n260 = call "Log error API.vi"("Error In"=w666) -> ("Error Out"=w668:errorcluster)  [unwired: 10 in]
              }
            }
          }
          frame True {
            n261 = call <vilib>:"Simple Error Handler.vi"("error in (no error)"=w669) -> ()  [unwired: 4 in, 5 out]
          }
        }
      }
    }
    "Config out" <- w26
  }
  "Error Out" <- w12
